vi "temp. meas. version2 v2_LV2010GF.vi"() -> ()   [LabVIEW 2010]
uses:
  Instance          15 36Saved   temp. meas. version2 v2 -jrb .vi
  Instance          16 36Saved   temp. meas. version2 v2 -jrb .vi
  Instance          17 36Saved   temp. meas. version2 v2 -jrb .vi
  Instance          18 36Saved   temp. meas. version2 v2 -jrb .vi
  Instance          19 36Saved   temp. meas. version2 v2 -jrb .vi
  Instance          20 36Saved   temp. meas. version2 v2 -jrb .vi
  <vilib>/Utility/file.llb/Read From Spreadsheet File (DBL).vi
  Instance           9 36Saved   temp. meas. version2 v2 -jrb .vi
  Instance          10 36Saved   temp. meas. version2 v2 -jrb .vi
  Instance          11 36Saved   temp. meas. version2 v2 -jrb .vi
  Instance          12 36Saved   temp. meas. version2 v2 -jrb .vi
  Instance          13 36Saved   temp. meas. version2 v2 -jrb .vi
  Instance          14 36Saved   temp. meas. version2 v2 -jrb .vi
  <vilib>/Utility/file.llb/Write To Spreadsheet File (DBL).vi
  <vilib>/Analysis/NI_AALBase.lvlib
panel:
  in  "Read Volt From Pi":bool=TRUE
  out "Voltage":string
  out "RPi temp2":string
  out "RPi Top Temp":string
  in  "Port":dbl=8901.0
  in  "IP Address":string="152.1.52.40"
  in  "Read Temp From Pi":bool=TRUE
  out "Laser Amp. Graph":cluster{"all rows":dbl[], "all rows":dbl[]}[](graph)=[{"all rows"=[32.91406, 52.36328, 73.22656, 93.29297, 112.7578], "all rows"=[-0.4725, -0.465, -0.4825, -0.485, -0.49]}]
  out "Paused":bool
  in  "NOTES":string
  in  "PAUSE next quasi wattime":bool
  in  "Num points to sum":i32=4
  out "Tive Vs Quasi-waittime*->":cluster{dbl[], dbl[]}[](graph)
  in  "PAUSE next ratio":bool
  in  "manually added info":T1
  out "lockin units":string
  out "Time v. counts/Las.Amp Graph":cluster{"all rows":dbl[], "all rows":dbl[]}[](graph)=[{"all rows"=[32.91406, 52.36328, 73.22656, 93.29297, 112.7578], "all rows"=[4.0, inf, -1.0, nan, 2.0]}]
  out "Gabes std (counter":dbl=nan format="%.3e"
  in  "Lockin settings":T2={"slope"=1, "Input Mode"=0, "time constant"=6, "display type"=1, "Range"=7, "Line reject"=1, "Filter Type"=0, "Auto freq tuning"=TRUE, "Filter Frequency (Hz)"=1000.0, "Auto Sensitivity"=FALSE, "Auto Measure"=FALSE, "Auto Phase"=TRUE} {"Filter Frequency (Hz)" min=2.0 max=1250000.0 step=1.0; "Filter Type" items=["Flat", "Notch", "Low-Pass", "Bandpass"]; "Line reject" items=["OFF", "2F", "F", "F & 2F"]; "Range" items=["100 nV", "300 nV", "1 uV", "3 uV", "10 uV", "30 uV", "100 uV", "300 uV", "1 mV", "3 mV", "10 mV", "30 mV", "100 mV", "300 mV", "1 V", "3 V"]; "display type" items=["Output %", "Output calibrated ", "Ratio", "log Ratio", "ADC 1", "ADC 2", " ADC 3", "ADC 4", "Noise %", "Noise Calibrated", "Ref. Frequency"]; "time constant" items=["1 ms", "3 ms", "10 ms", "30 ms", "100 ms", "300 ms", "1 s", "3 s", "10 s", "30 s", "100 s", "300 s", "1 ks", "3 ks"]; "Input Mode" items=["Voltage Input ( A or A-B)", "Current Input 10E6 V/A", "Current Input 10E8 V/A"]; "slope" items=["6dB/octave", "12dB/octave"]}
  out "Extra Steps taken DOWN":dbl
  out "Extra Steps taken UP":dbl
  in  "Extra steps on way TO TROUGH":dbl
  in  "extra steps on way TO PEAK":dbl
  out "peak loop counter":u32=1
  out "trough loop counter":u32=1
  out "lockin peak std":dbl=0.0050000000000000044
  out "lockin peak avg.":dbl=-0.495
  out "cB peak std":dbl=0.5
  out "cB peak avg.":dbl=0.5
  out "cA peak std":dbl
  out "cA peak avg.":dbl
  out "lockin  trough std":dbl=0.0050000000000000044
  out "lockin  trough avg.":dbl=-0.485
  out "cB trough std":dbl=1.0
  out "cB  trough avg":dbl=1.0
  out "cA trough std":dbl
  out "cA trough avg.":dbl
  in  "(m) # measurements \npe r wavelength":dbl=1.0 format="%#_2f"
  out "Time v. Ratio Graph":cluster{"all rows":dbl[], "all rows":dbl[]}[](graph)=[{"all rows"=[32.91406, 52.36328, 73.22656, 93.29297, 112.7578], "all rows"=[4.0, inf, -1.0, nan, 2.0]}]
  in  "Current Wavelength (nm)":dbl=475.0
  in  "GPIB Address SR400":string="0:23"
  in  "File name (all data)":string="temp_stats.txt"
  in  "File path":path=path "C:/users/Data/fluorescence"
  out "Ratio (counter)":dbl=2.0 format="%.3e"
  out "std (counter)":dbl=nan format="%.3e"
  out "std":dbl=4.817177617164692 format="%.3e"
  out "Time":dbl=112.7578125 format="%.3e"
  out "meas. loop counter (0 to n-1)":u32=4
  in  "# Temp. Meas. (n)":i32=10000
  out "std (lockin)":dbl=-0.00500078099915926 format="%.2f"
  out "Laser Amp. (lockin)":dbl=-0.49 format="%.3e"
  out "peak wavelength":i32=474 format="%.1f"
  out "peak lockin":dbl=-0.5 format="%.4e"
  out "peak counter B":dbl format="%.4e"
  out "peak counter A":dbl format="%.4e"
  in  "Start Wavelength (nm)":dbl=475.0
  out "trough wavelength":i32=460 format="%.1f"
  out "trough lockin":dbl=-0.48 format="%.4e"
  out "trough counter B":dbl format="%.4e"
  out "trough counter A":dbl format="%.4e"
  in  "Mode Control":T3(ring)
  in  "Wait Time (s)":dbl=5.0
  in  "Peak Wavelength (nm)":dbl=475.0
  in  "Trough Wavelength (nm)":dbl=465.0
  out "Wavelength Range Warning":bool
  in  "GPIB Address Lock-In":u8=12 min=1 max=32 step=1
  in  "GPIB Address OSC (GPIB[1]::4)":string="GPIB0::4"
  in  "Parallel Port Address":i16=888 format="%.0x"
  # "GABRIELS VARIANT OF Temperature Fluorescence Measurement"
  # "This program uses the first GPIB board (GPIB0)\ndefault addresses:\n     monochromator   x378 (parallel port)\n     lockin  GPIB0::12 (hardwired\n     osc      GPIB0::4 (not used)\n     counter 0:23"
  # "Oscilloscope Setup\n(TEKTRONIX TDS 420)"
  # "Photon Counter Setup\n(SRS 400)"
  # "Monochromator Setup\n(SPEX 1680B)"
  # "Lock-In Setup\n(EG&G 5209)"
  # "Perylene**: wavelength pairs: literature 464/476 nm \n                                             measured*: 460/475 nm\n                       ckc measured (Mar 2014): 464/476 nm"
  # "Gabes Variant"
  # "LAST DATA POINT"
  # "LAST TEMP. MEASUREMENT"
  # "**  A. J. Bur, M. G. Vangel, and S. Roth \"Temperature Dependence of Fluorescent Probes\nfor Applications to Polymer Materials Processing,\" Appl. Spec. 56, 174 (2002)."
  # "EG&G 5209 Lockin Amplifier:\n1. Manually set appropriate front\npanel settings (Sensitivity, Filters,\nand Phase).\n2. Set Time Constant to be appropriate for\nthe given REF FREQ and Wait Time (used\nabove)."
  # "SR400 Photon Counter:\n1. Run photon counter vi\nor manually control desired\nsettings.\n2. Set Wait Time to Tpreset\n3. Run this program."
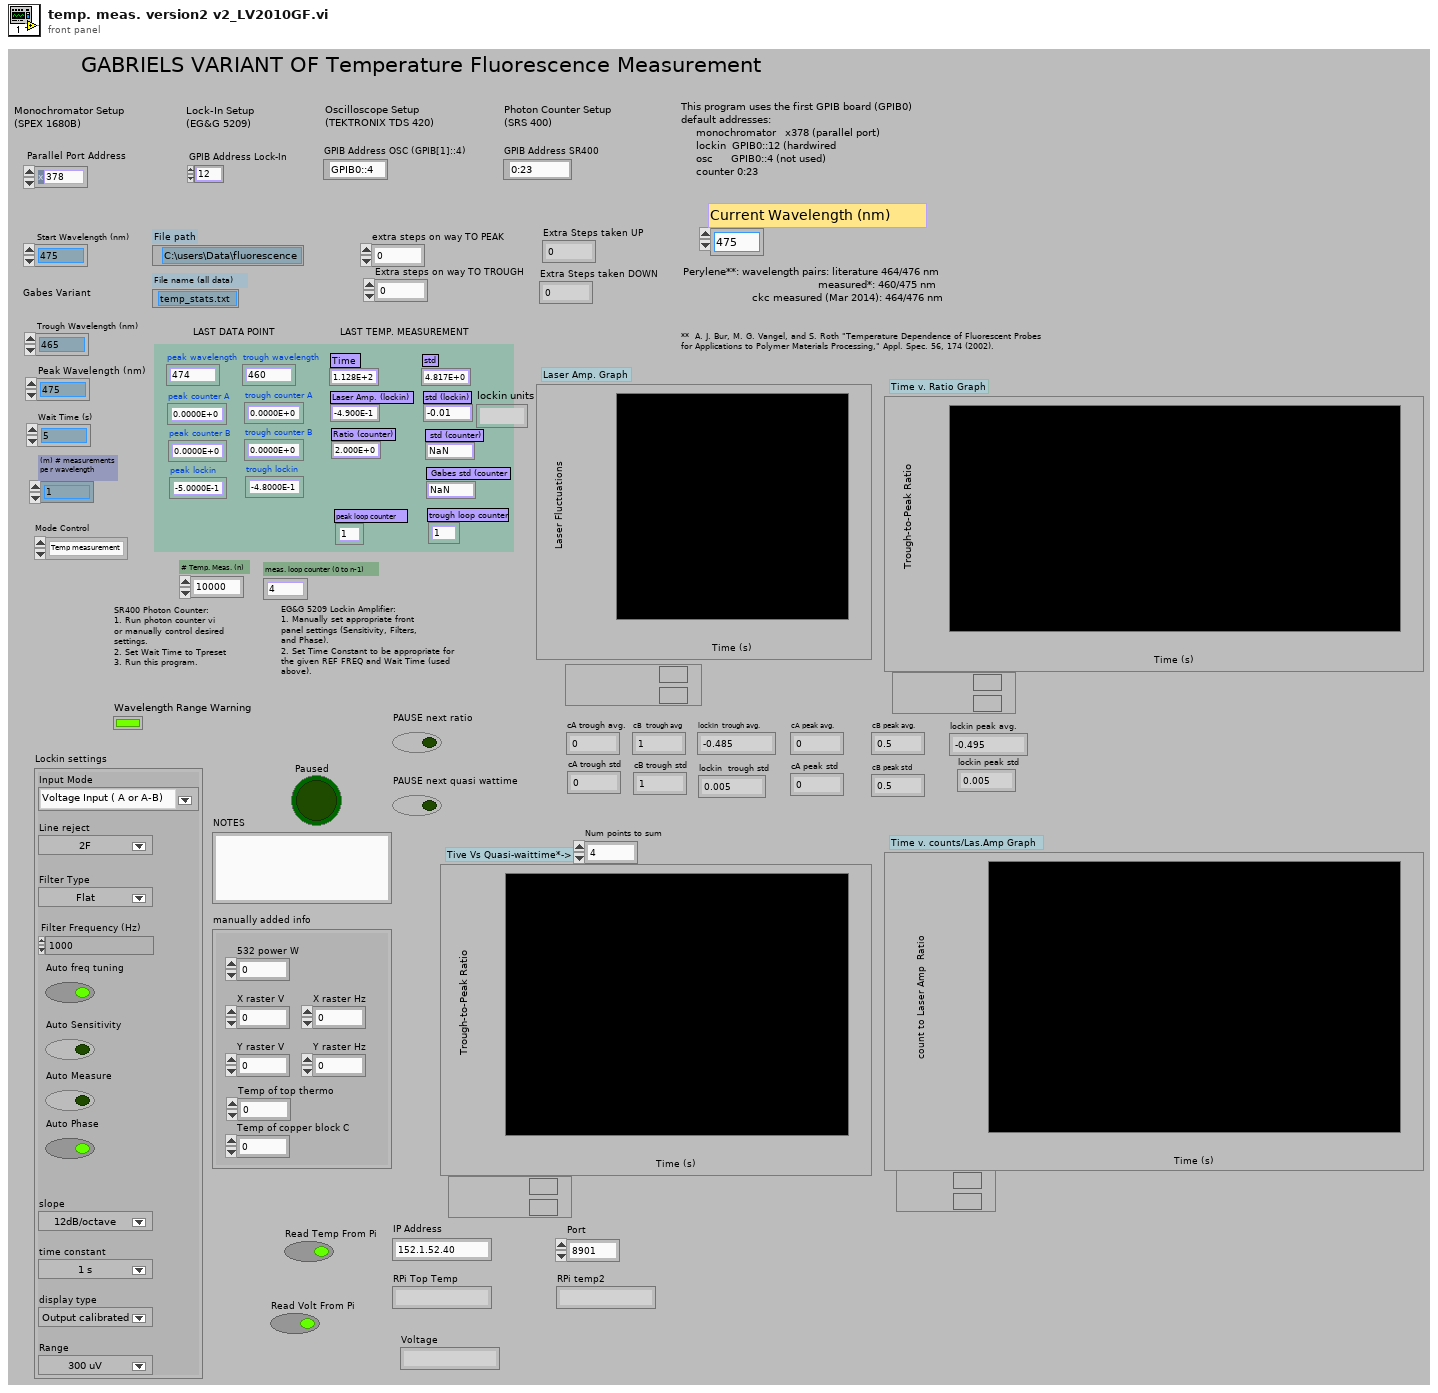
[diagram p1: front panel]
types:
  T1 = cluster{"532 power W":dbl, "X raster V":dbl, "X raster Hz ":dbl, "Y raster V":dbl, "Y raster Hz":dbl, "Temp of copper block C":dbl, "Temp of top thermo":dbl}
  T2 = cluster{"slope":i32, "Input Mode":i32, "time constant":i32, "display type":i32, "Range":i32, "Line reject":i32, "Filter Type":i32, "Auto freq tuning":bool, "Filter Frequency (Hz)":dbl, "Auto Sensitivity":bool, "Auto Measure":bool, "Auto Phase":bool}
  T3 = enum32{"Temp measurement", "Temperature Measurement"}
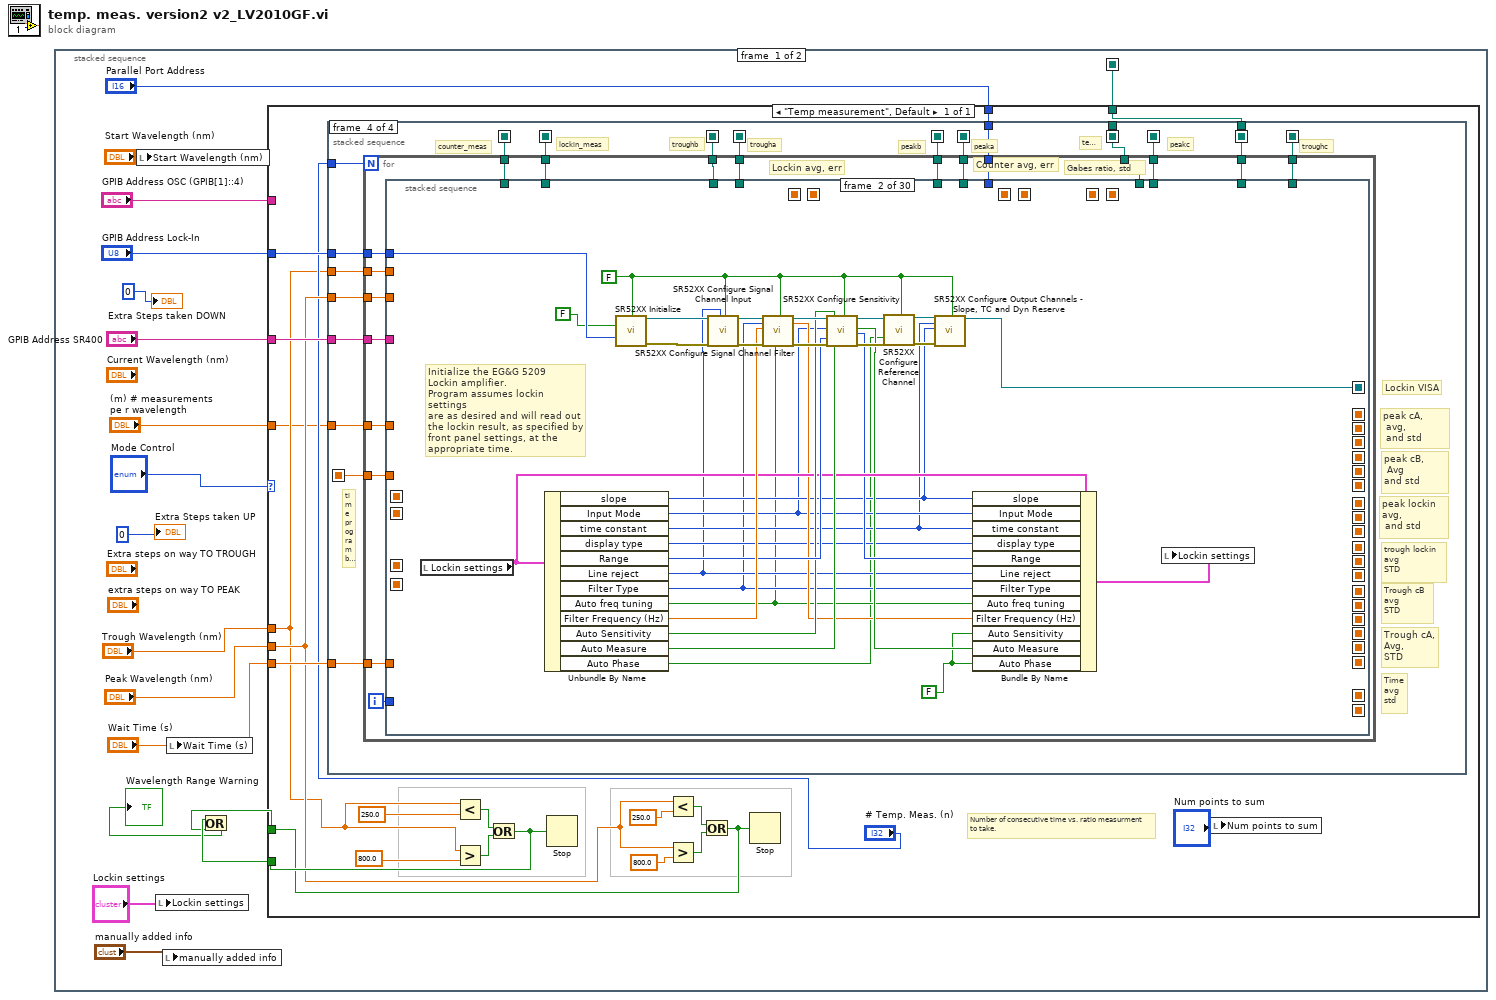
[diagram p0: block diagram]
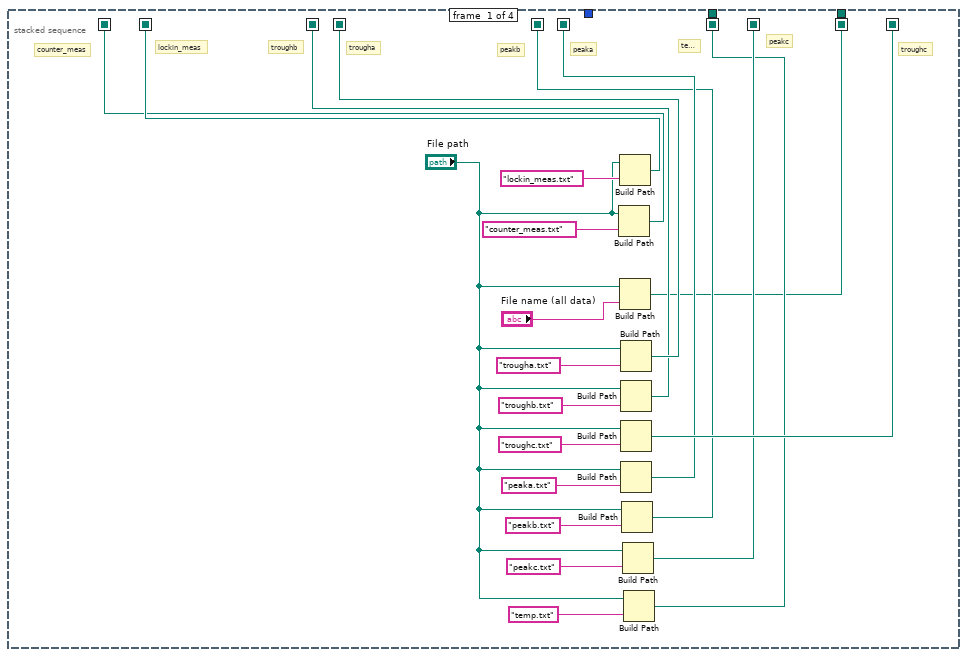
[diagram p2: hidden frame]
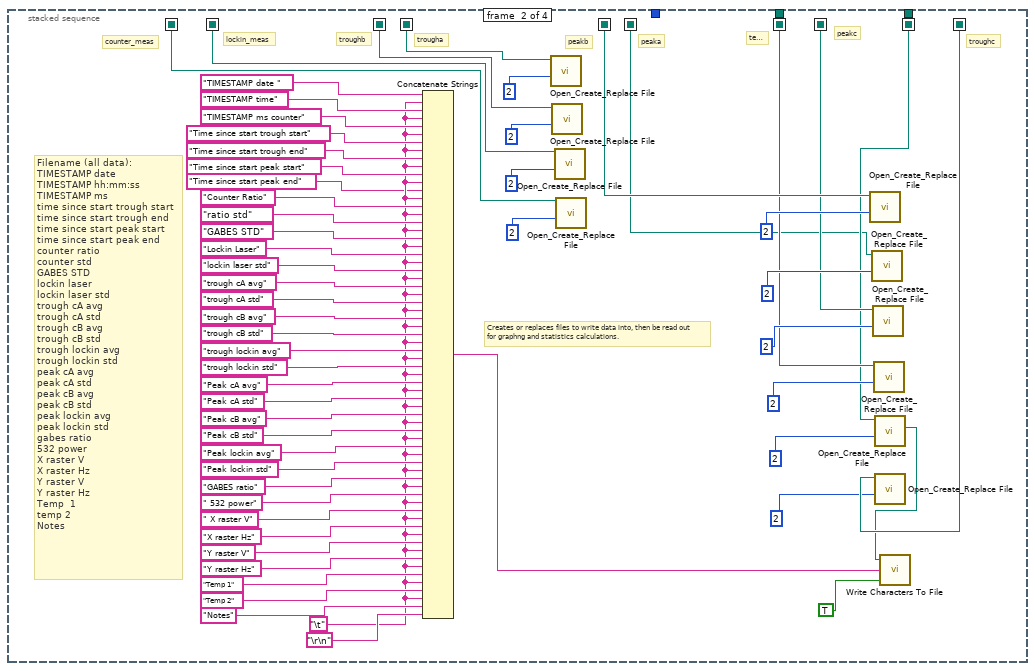
[diagram p3: hidden frame]
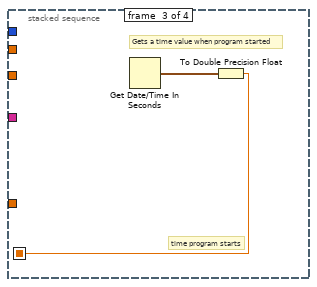
[diagram p4: hidden frame]
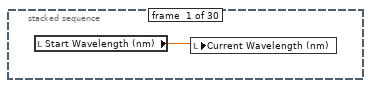
[diagram p5: hidden frame]
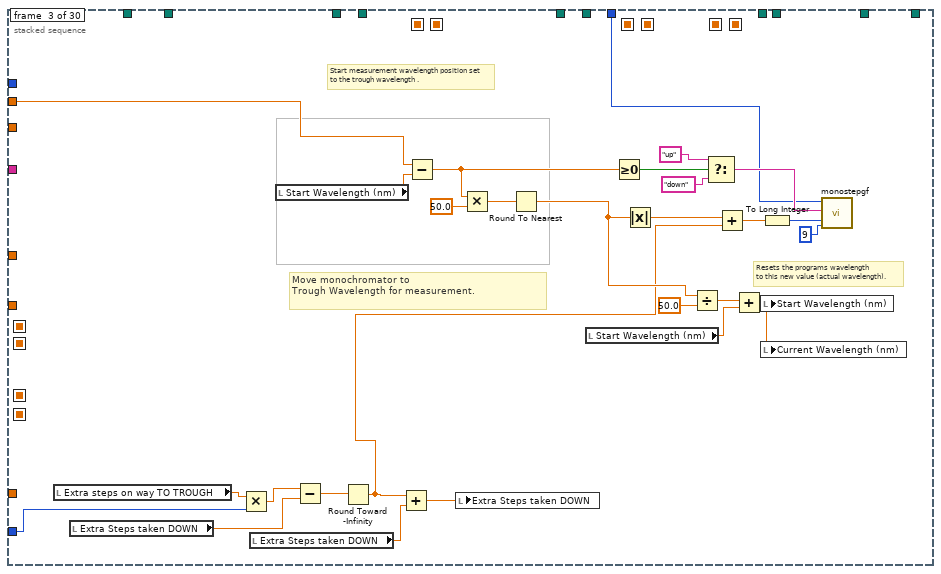
[diagram p6: hidden frame]
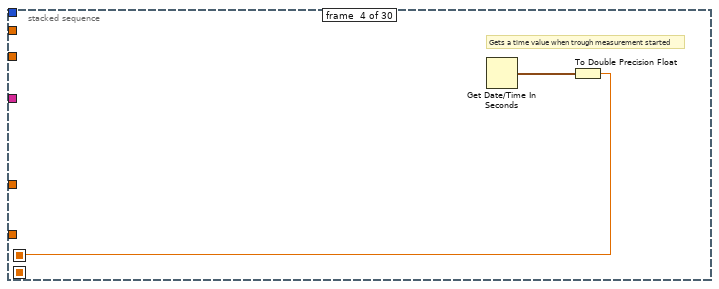
[diagram p7: hidden frame]
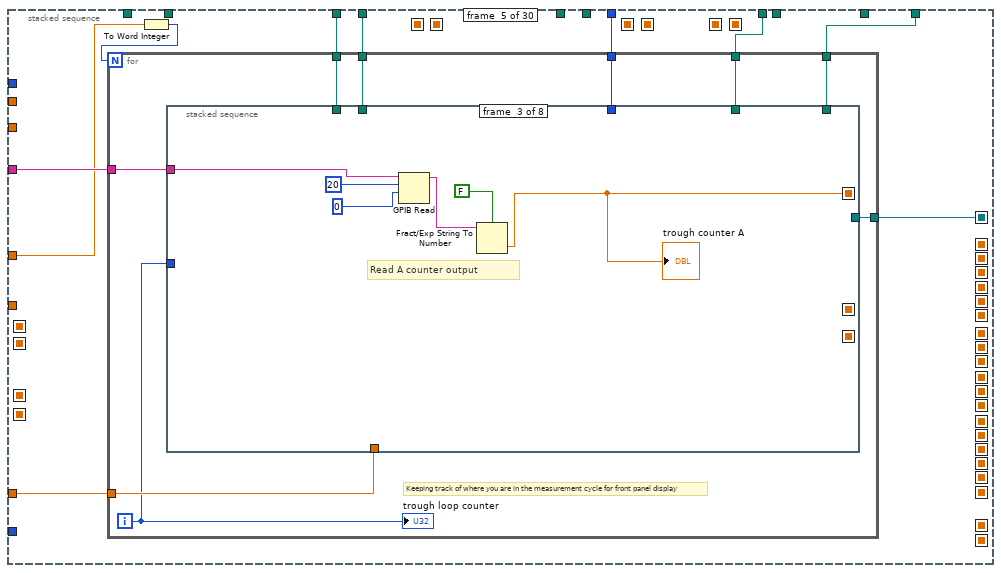
[diagram p8: hidden frame]
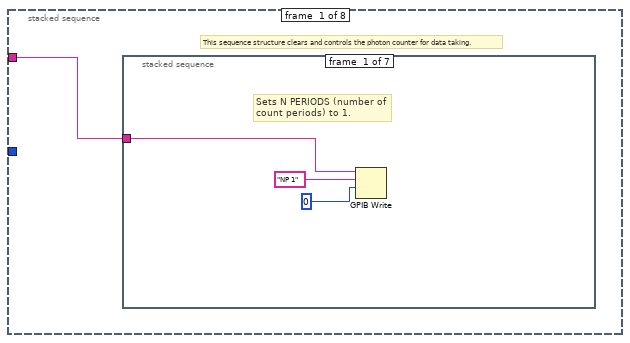
[diagram p9: hidden frame]
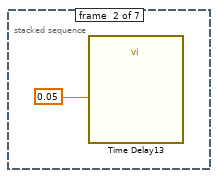
[diagram p10: hidden frame]
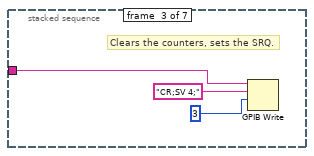
[diagram p11: hidden frame]
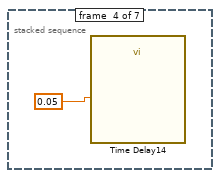
[diagram p12: hidden frame]
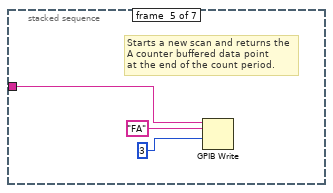
[diagram p13: hidden frame]
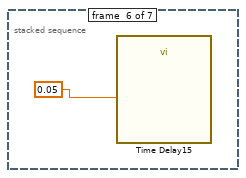
[diagram p14: hidden frame]
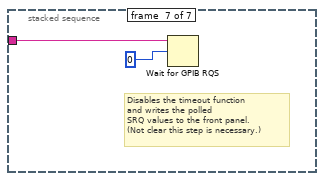
[diagram p15: hidden frame]
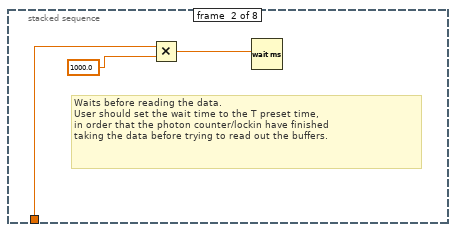
[diagram p16: hidden frame]
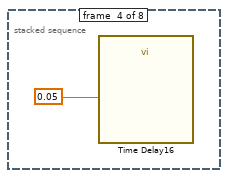
[diagram p17: hidden frame]
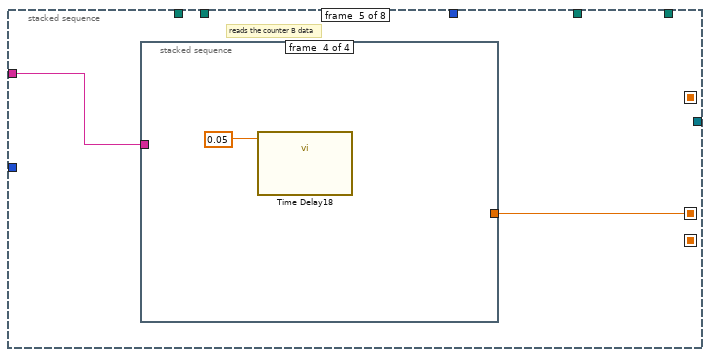
[diagram p18: hidden frame]
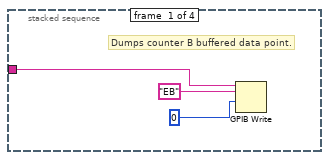
[diagram p19: hidden frame]
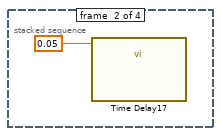
[diagram p20: hidden frame]
diagram:
  n1 = stacked-sequence {
    seq-local: [w10 _] -> [_ w887]
    frame #0 {
      n2 = local write "Start Wavelength (nm)"("Start Wavelength (nm)") -> ()
      n3 = local write "Lockin settings"("Lockin settings") -> ()
      n4 = local write "manually added info"("manually added info") -> ()
      n5 = local write "Wait Time (s)"("Wait Time (s)") -> ()
      n6 = case shown="\"Temp measurement\", Default" "Mode Control" {
        tunnel: "Parallel Port Address" -> [w30]
        tunnel: "GPIB Address OSC (GPIB[1]::4)" -> [_]
        tunnel: [w26] -> w16
        tunnel: [w24] -> w15
        tunnel: "GPIB Address Lock-In" -> [w27]
        tunnel: "GPIB Address SR400" -> [w29]
        tunnel: "Peak Wavelength (nm)" -> [w25]
        tunnel: "Trough Wavelength (nm)" -> [w22]
        tunnel: "Wait Time (s)" -> [w28]
        tunnel: [w20] -> w10
        tunnel: "(m) # measurements \npe r wavelength" -> [w21]
        frame "Temp measurement", Default {
          # "Number of consecutive time vs. ratio measurment\nto take."
          n7 = stacked-sequence {
            seq-local: [_ _ w118 _] -> [_ _ _ w131]
            seq-local: [w59 _ _ _] -> [_ w75 _ w130]
            seq-local: [w41 _ _ _] -> [_ w104 _ w129]
            seq-local: [w50 _ _ _] -> [_ w76 _ w127]
            seq-local: [w51 _ _ _] -> [_ w73 _ w128]
            seq-local: [w49 _ _ _] -> [_ w117 _ w126]
            seq-local: [w47 _ _ _] -> [_ w107 _ w124]
            seq-local: [w48 _ _ _] -> [_ w102 _ w125]
            seq-local: [w46 _ _ _] -> [_ w105 _ w123]
            seq-local: [w44 _ _ _] -> [_ w106 _ w122]
            seq-local: [w39 _ _ _] -> [_ w74 _ w121]
            tunnel: w22 -> [_ _ _ w138]
            tunnel: w30 -> [_ _ _ w137]
            tunnel: w25 -> [_ _ _ w133]
            tunnel: w29 -> [_ _ _ w134]
            tunnel: w27 -> [_ _ _ w136]
            tunnel: w28 -> [_ _ _ w135]
            tunnel: "# Temp. Meas. (n)" -> [_ _ _ w132]
            tunnel: [w44 _ _ _] -> _
            tunnel: w21 -> [_ _ _ w120]
            tunnel: [w41 _ _ _] -> w20
            frame #0 {
              # "temp"
              # "counter_meas"
              # "lockin_meas"
              # "peakc"
              # "peakb"
              # "peaka"
              # "troughc"
              # "troughb"
              # "trougha"
              n8 = Build Path(base path="File path", name or relative path="counter_meas.txt") -> (appended path=w39:path)
              n9 = Build Path(base path="File path", name or relative path="lockin_meas.txt") -> (appended path=w59:path)
              n10 = Build Path(base path="File path", name or relative path="File name (all data)") -> (appended path=w41:path)
              n11 = Build Path(base path="File path", name or relative path="trougha.txt") -> (appended path=w51:path)
              n12 = Build Path(base path="File path", name or relative path="troughb.txt") -> (appended path=w50:path)
              n13 = Build Path(base path="File path", name or relative path="troughc.txt") -> (appended path=w49:path)
              n14 = Build Path(base path="File path", name or relative path="peaka.txt") -> (appended path=w48:path)
              n15 = Build Path(base path="File path", name or relative path="peakb.txt") -> (appended path=w47:path)
              n16 = Build Path(base path="File path", name or relative path="peakc.txt") -> (appended path=w46:path)
              n17 = Build Path(base path="File path", name or relative path="temp.txt") -> (appended path=w44:path)
            }
            frame #1 {
              w61 = "\t"
              # "temp"
              # "counter_meas"
              # "lockin_meas"
              # "peakc"
              # "peakb"
              # "peaka"
              # "troughc"
              # "troughb"
              # "trougha"
              # "Filename (all data):\nTIMESTAMP date\nTIMESTAMP hh:mm:ss\nTIMESTAMP ms\ntime since start trough start\ntime since start trough end\ntime since start peak start\ntime since start peak end\ncounter ratio\ncounter std\nGABES STD\nlockin laser\nlockin laser std\ntrough cA avg\ntrough cA std\ntrough cB avg\ntrough cB std\ntrough lockin avg\ntrough lockin std\npeak cA avg\npeak cA std\npeak cB avg\npeak cB std\npeak lockin avg\npeak lockin std\ngabes ratio\n532 power\nX raster V\nX raster Hz\nY raster V\nY raster Hz\nTemp  1\ntemp 2\nNotes"
              # "Creates or replaces files to write data into, then be read out\nfor graphng and statistics calculations."
              n18 = Concatenate Strings("TIMESTAMP date ", w61, "TIMESTAMP time", w61, "TIMESTAMP ms counter", w61, "Time since start trough start", w61, "Time since start trough end", w61, "Time since start peak start", w61, "Time since start peak end", w61, "Counter Ratio", w61, "ratio std", w61, "GABES STD", w61, "Lockin Laser", w61, "lockin laser std", w61, "trough cA avg", w61, "trough cA std", w61, "trough cB avg", w61, "trough cB std", w61, "trough lockin avg", w61, "trough lockin std", w61, "Peak cA avg", w61, "Peak cA std", w61, "Peak cB avg", w61, "Peak cB std", w61, "Peak lockin avg", w61, "Peak lockin std", w61, "GABES ratio", w61, " 532 power", w61, " X raster V", w61, "X raster Hz", w61, "Y raster V", w61, "Y raster Hz", w61, "Temp 1", w61, "Temp 2", w61, "Notes", "\r\n") -> (w83:string)
              n19 = call <vilib>:"Open_Create_Replace File.vi"("function (open:0)"=2, "file path"=w73) -> ()  [unwired: 6 in, 4 out]
              n20 = call <vilib>:"Open_Create_Replace File.vi"("function (open:0)"=2, "file path"=w76) -> ()  [unwired: 6 in, 4 out]
              n21 = call <vilib>:"Open_Create_Replace File.vi"("function (open:0)"=2, "file path"=w75) -> ()  [unwired: 6 in, 4 out]
              n22 = call <vilib>:"Open_Create_Replace File.vi"("function (open:0)"=2, "file path"=w74) -> ()  [unwired: 6 in, 4 out]
              n23 = call <vilib>:"Open_Create_Replace File.vi"("function (open:0)"=2, "file path"=w107) -> ()  [unwired: 6 in, 4 out]
              n24 = call <vilib>:"Open_Create_Replace File.vi"("function (open:0)"=2, "file path"=w102) -> ()  [unwired: 6 in, 4 out]
              n25 = call <vilib>:"Open_Create_Replace File.vi"("function (open:0)"=2, "file path"=w105) -> ()  [unwired: 6 in, 4 out]
              n26 = call <vilib>:"Open_Create_Replace File.vi"("function (open:0)"=2, "file path"=w106) -> ()  [unwired: 6 in, 4 out]
              n27 = call <vilib>:"Open_Create_Replace File.vi"("function (open:0)"=2, "file path"=w104) -> ("new file path"=w82:path)  [unwired: 6 in, 3 out]
              n28 = call <vilib>:"Open_Create_Replace File.vi"("function (open:0)"=2, "file path"=w117) -> ()  [unwired: 6 in, 4 out]
              n29 = call <vilib>:"Write Characters To File.vi"("append to file? (new file:F)"=TRUE, "character string"=w83, "file path (dialog if empty)"=w82) -> ()  [unwired: 2 in, 1 out]
            }
            frame #2 {
              # "time program starts"
              # "Gets a time value when program started"
              n30 = Get Date/Time In Seconds() -> (seconds since 1Jan1904=w119:timestamp)
              n31 = To Double Precision Float(number=w119) -> (double precision float=w118:dbl)
            }
            frame #3 {
              # "time program began"
              # "Trough cA,\nAvg,\nSTD"
              # "Time\navg\nstd"
              # "trough lockin\navg\nSTD"
              # "Trough cB\navg\nSTD"
              # "Lockin VISA"
              # "peak cB,\n Avg\nand std"
              # "peak cA,\n avg,\n and std"
              # "peak lockin  avg,\n and std"
              # "temp"
              # "counter_meas"
              # "lockin_meas"
              # "peakc"
              # "peakb"
              # "peaka"
              # "troughc"
              # "troughb"
              # "trougha"
              n32 = for {
                N: w132 -> [_]
                tunnel: w138 -> [w157]
                tunnel: w137 -> [w156]
                tunnel: w136 -> [w155]
                tunnel: w135 -> [w154]
                tunnel: w134 -> [w153]
                tunnel: w133 -> [w152]
                tunnel: w131 -> [w150]
                tunnel: w130 -> [w149]
                tunnel: w129 -> [w148]
                tunnel: w128 -> [w147]
                tunnel: w127 -> [w146]
                tunnel: w126 -> [w145]
                tunnel: w125 -> [w144]
                tunnel: w124 -> [w143]
                tunnel: w123 -> [w142]
                tunnel: w122 -> [w141]
                tunnel: w121 -> [w140]
                tunnel: w120 -> [w139]
                i -> [w151]
                # "Gabes ratio, std"
                # "Counter avg, err"
                # "Lockin avg, err"
                n33 = stacked-sequence {
                  seq-local: [_ w174 _ _ _ _ _ _ _ _ _ _ _ _ _ _ _ _ _ _ _ _ _ _ _ _ _ _ _ _] -> [_ _ _ _ w226 _ _ _ _ _ _ _ _ w427 _ _ _ _ _ _ _ _ _ _ _ _ _ _ _ w855]
                  seq-local: [_ _ _ _ _ _ _ w318 _ _ _ _ _ _ _ _ _ _ _ _ _ _ _ _ _ _ _ _ _ _] -> [_ _ _ _ _ _ _ _ _ _ _ _ _ _ _ _ _ _ _ _ _ w615 _ w660 w717 _ _ _ _ _]
                  seq-local: [_ _ _ _ _ _ _ w317 _ _ _ _ _ _ _ _ _ _ _ _ _ _ _ _ _ _ _ _ _ _] -> [_ _ _ _ _ _ _ _ _ _ _ _ _ _ _ _ _ _ _ _ _ w621 _ w661 w718 _ _ _ _ _]
                  seq-local: [_ _ _ _ _ _ _ _ w323 _ _ _ _ _ _ _ _ _ _ _ _ _ _ _ _ _ _ _ _ _] -> [_ _ _ _ _ _ _ _ _ _ _ _ _ _ _ _ _ _ _ _ _ w613 _ w659 w715 _ _ _ _ _]
                  seq-local: [_ _ _ _ _ _ _ _ w324 _ _ _ _ _ _ _ _ _ _ _ _ _ _ _ _ _ _ _ _ _] -> [_ _ _ _ _ _ _ _ _ _ _ _ _ _ _ _ _ _ _ _ _ w620 _ w658 w716 _ _ _ _ _]
                  seq-local: [_ _ _ _ _ _ _ _ _ w329 _ _ _ _ _ _ _ _ _ _ _ _ _ _ _ _ _ _ _ _] -> [_ _ _ _ _ _ _ _ _ _ _ _ _ _ _ _ _ _ _ _ w588 _ _ _ w713 _ _ _ _ _]
                  seq-local: [_ _ _ _ _ _ _ _ _ w330 _ _ _ _ _ _ _ _ _ _ _ _ _ _ _ _ _ _ _ _] -> [_ _ _ _ _ _ _ _ _ _ _ _ _ _ _ _ _ _ _ _ w587 _ _ _ w714 _ _ _ _ _]
                  seq-local: [_ _ _ _ _ _ _ _ _ _ _ _ _ _ _ _ _ _ _ w564 _ _ _ _ _ _ _ _ _ _] -> [_ _ _ _ _ _ _ _ _ _ _ _ _ _ _ _ _ _ _ _ _ _ _ _ _ _ _ _ _ _]
                  seq-local: [_ _ _ _ _ _ _ _ _ _ _ _ _ _ _ _ _ _ _ w563 _ _ _ _ _ _ _ _ _ _] -> [_ _ _ _ _ _ _ _ _ _ _ _ _ _ _ _ _ _ _ _ _ _ _ _ _ w740 _ _ _ _]
                  seq-local: [_ _ _ _ _ _ _ _ _ _ _ _ _ _ _ _ _ w553 _ _ _ _ _ _ _ _ _ _ _ _] -> [_ _ _ _ _ _ _ _ _ _ _ _ _ _ _ _ _ _ _ _ _ w619 _ w680 w707 _ _ _ _ _]
                  seq-local: [_ _ _ _ _ _ _ _ _ _ _ _ _ _ _ _ _ w552 _ _ _ _ _ _ _ _ _ _ _ _] -> [_ _ _ _ _ _ _ _ _ _ _ _ _ _ _ _ _ _ _ _ _ w623 _ w676 w708 _ _ _ _ _]
                  seq-local: [_ _ _ _ _ _ _ _ _ _ _ _ _ _ _ _ _ _ w559 _ _ _ _ _ _ _ _ _ _ _] -> [_ _ _ _ _ _ _ _ _ _ _ _ _ _ _ _ _ _ _ _ _ w617 _ w679 w709 _ _ _ _ _]
                  seq-local: [_ _ _ _ _ _ _ _ _ _ _ _ _ _ _ _ _ _ w558 _ _ _ _ _ _ _ _ _ _ _] -> [_ _ _ _ _ _ _ _ _ _ _ _ _ _ _ _ _ _ _ _ _ w622 _ w672 w710 _ _ _ _ _]
                  seq-local: [_ _ _ _ _ _ _ _ _ _ _ _ _ _ _ _ w547 _ _ _ _ _ _ _ _ _ _ _ _ _] -> [_ _ _ _ _ _ _ _ _ _ _ _ _ _ _ _ _ _ _ _ w598 _ _ _ w711 _ _ _ _ _]
                  seq-local: [_ _ _ _ _ _ _ _ _ _ _ _ _ _ _ _ w546 _ _ _ _ _ _ _ _ _ _ _ _ _] -> [_ _ _ _ _ _ _ _ _ _ _ _ _ _ _ _ _ _ _ _ w597 _ _ _ w712 _ _ _ _ _]
                  seq-local: [_ _ _ w218 _ _ _ _ _ _ _ _ _ _ _ _ _ _ _ _ _ _ _ _ _ _ _ _ _ _] -> [_ _ _ _ _ _ _ _ _ _ _ _ _ _ _ _ _ _ _ w568 _ _ _ _ w688 _ _ _ _ _]
                  seq-local: [_ _ _ _ _ _ w314 _ _ _ _ _ _ _ _ _ _ _ _ _ _ _ _ _ _ _ _ _ _ _] -> [_ _ _ _ _ _ _ _ _ _ _ _ _ _ _ _ _ _ _ w567 _ _ _ _ w687 _ _ _ _ _]
                  seq-local: [_ _ _ _ _ _ _ _ _ _ _ _ w419 _ _ _ _ _ _ _ _ _ _ _ _ _ _ _ _ _] -> [_ _ _ _ _ _ _ _ _ _ _ _ _ _ _ _ _ _ _ w566 _ _ _ _ w686 _ _ _ _ _]
                  seq-local: [_ _ _ _ _ _ _ _ _ _ _ _ _ _ w515 _ _ _ _ _ _ _ _ _ _ _ _ _ _ _] -> [_ _ _ _ _ _ _ _ _ _ _ _ _ _ _ _ _ _ _ w565 _ _ _ _ w685 _ _ _ _ _]
                  seq-local: [_ _ _ _ _ _ _ _ _ _ _ _ _ _ _ _ _ _ _ _ w589 _ _ _ _ _ _ _ _ _] -> [_ _ _ _ _ _ _ _ _ _ _ _ _ _ _ _ _ _ _ _ _ _ _ _ w734 w748 _ _ _ _]
                  seq-local: [_ _ _ _ _ _ _ _ _ _ _ _ _ _ _ _ _ _ _ _ w596 _ _ _ _ _ _ _ _ _] -> [_ _ _ _ _ _ _ _ _ _ _ _ _ _ _ _ _ _ _ _ _ _ _ _ w735 _ _ _ _ _]
                  seq-local: [_ _ _ _ _ _ _ _ _ _ _ _ _ _ _ _ _ _ _ _ _ w610 _ _ _ _ _ _ _ _] -> [_ _ _ _ _ _ _ _ _ _ _ _ _ _ _ _ _ _ _ _ _ _ _ _ w690 w742 _ _ _ _]
                  seq-local: [_ _ _ _ _ _ _ _ _ _ _ _ _ _ _ _ _ _ _ _ _ w609 _ _ _ _ _ _ _ _] -> [_ _ _ _ _ _ _ _ _ _ _ _ _ _ _ _ _ _ _ _ _ _ _ _ w732 _ _ _ _ _]
                  seq-local: [_ _ _ _ _ _ _ _ _ _ _ _ _ _ _ _ _ _ _ _ _ _ _ w678 _ _ _ _ _ _] -> [_ _ _ _ _ _ _ _ _ _ _ _ _ _ _ _ _ _ _ _ _ _ _ _ w706 _ _ _ _ _]
                  seq-local: [_ _ _ _ _ _ _ _ _ _ _ _ _ _ _ _ w545 _ _ _ _ _ _ _ _ _ _ _ _ _] -> [_ _ _ _ _ _ _ _ _ _ _ _ _ _ _ _ _ _ _ _ _ _ w644 _ _ _ _ _ _ _]
                  seq-local: [_ _ _ _ _ _ _ _ _ w328 _ _ _ _ _ _ _ _ _ _ _ _ _ _ _ _ _ _ _ _] -> [_ _ _ _ _ _ _ _ _ _ _ _ _ _ _ _ _ _ _ _ _ _ w642 _ _ _ _ _ _ _]
                  seq-local: [_ _ _ _ _ _ _ _ w322 _ _ _ _ _ _ _ _ _ _ _ _ _ _ _ _ _ _ _ _ _] -> [_ _ _ _ _ _ _ _ _ _ _ _ _ _ _ _ _ _ _ _ _ _ w645 _ _ _ _ _ _ _]
                  seq-local: [_ _ _ _ _ _ _ _ _ _ _ _ _ _ _ _ _ w551 _ _ _ _ _ _ _ _ _ _ _ _] -> [_ _ _ _ _ _ _ _ _ _ _ _ _ _ _ _ _ _ _ _ _ _ w647 _ _ _ _ _ _ _]
                  seq-local: [_ _ _ _ _ _ _ _ _ _ _ _ _ _ _ _ _ _ w557 _ _ _ _ _ _ _ _ _ _ _] -> [_ _ _ _ _ _ _ _ _ _ _ _ _ _ _ _ _ _ _ _ _ _ w646 _ _ _ _ _ _ _]
                  seq-local: [_ _ _ _ _ _ _ _ _ _ _ _ _ _ _ _ _ _ _ _ _ _ w638 _ _ _ _ _ _ _] -> [_ _ _ _ _ _ _ _ _ _ _ _ _ _ _ _ _ _ _ _ _ _ _ _ w719 w739 _ _ _ _]
                  seq-local: [_ _ _ _ _ _ _ w316 _ _ _ _ _ _ _ _ _ _ _ _ _ _ _ _ _ _ _ _ _ _] -> [_ _ _ _ _ _ _ _ _ _ _ _ _ _ _ _ _ _ _ _ _ _ w643 _ _ _ _ _ _ _]
                  tunnel: w157 -> [_ _ w202 _ _ _ _ _ _ _ _ _ _ _ _ _ _ _ _ _ _ _ _ _ _ _ _ _ _ _]
                  tunnel: w156 -> [_ _ w206 _ w227 _ _ _ _ _ _ w405 _ w428 _ _ _ _ _ _ _ _ _ _ _ _ _ _ _ _]
                  tunnel: w155 -> [_ w190 _ _ _ _ _ _ _ _ _ _ _ _ _ _ _ _ _ _ _ _ _ _ _ _ _ _ _ _]
                  tunnel: w154 -> [_ _ _ _ w229 _ _ _ _ _ _ _ _ w429 _ _ _ _ _ _ _ _ _ _ _ _ _ _ _ _]
                  tunnel: w153 -> [_ _ _ _ w228 _ _ _ _ _ _ _ _ w430 _ _ _ _ _ _ _ _ _ _ _ _ _ _ _ _]
                  tunnel: w152 -> [_ _ _ _ _ _ _ _ _ _ _ w403 _ _ _ _ _ _ _ _ _ _ _ _ _ _ _ _ _ _]
                  tunnel: w151 -> [_ _ w192 _ _ _ _ _ _ _ _ w393 _ _ _ _ _ _ _ _ w599 _ _ _ _ _ _ _ _ _]
                  tunnel: w150 -> [_ _ _ _ _ _ _ _ _ _ _ _ _ _ _ _ _ _ _ w569 _ _ _ _ w689 _ _ _ _ _]
                  tunnel: w149 -> [_ _ _ _ _ _ _ _ _ _ _ _ _ _ _ _ _ _ _ _ _ _ _ _ _ w747 _ _ _ _]
                  tunnel: w148 -> [_ _ _ _ _ _ _ _ _ _ _ _ _ _ _ _ _ _ _ _ _ _ _ _ w733 _ _ _ w797 _]
                  tunnel: w147 -> [_ _ _ _ w225 _ _ w319 _ _ _ _ _ _ _ _ _ _ _ _ _ _ _ _ _ _ _ _ _ w871]
                  tunnel: w146 -> [_ _ _ _ w224 _ _ _ w325 _ _ _ _ _ _ _ _ _ _ _ _ _ _ _ _ _ _ _ _ w870]
                  tunnel: w145 -> [_ _ _ _ w223 _ _ _ _ w331 _ _ _ _ _ _ _ _ _ _ _ _ _ _ _ _ _ _ _ w856]
                  tunnel: w144 -> [_ _ _ _ _ _ _ _ _ _ _ _ _ w426 _ _ _ w554 _ _ _ _ _ _ _ _ _ _ _ w862]
                  tunnel: w143 -> [_ _ _ _ _ _ _ _ _ _ _ _ _ w425 _ _ _ _ w560 _ _ _ _ _ _ _ _ _ _ w863]
                  tunnel: w142 -> [_ _ _ _ _ _ _ _ _ _ _ _ _ w424 _ _ w548 _ _ _ _ _ _ _ _ _ _ _ _ w857]
                  tunnel: w141 -> [_ _ _ _ w222 _ _ _ _ _ _ _ _ w423 _ _ _ _ _ _ _ _ _ _ _ _ _ _ _ _]
                  tunnel: w140 -> [_ _ _ _ _ _ _ _ _ _ _ _ _ _ _ _ _ _ _ _ _ _ _ _ _ w741 _ w759 _ _]
                  tunnel: w139 -> [_ _ _ _ w221 _ _ _ _ _ _ _ _ w422 _ _ _ _ _ _ _ _ _ _ _ _ _ _ _ _]
                  frame #0 {
                    n34 = local read "Start Wavelength (nm)"() -> (w158:dbl)
                    n35 = local write "Current Wavelength (nm)"(w158) -> ()
                  }
                  frame #1 {
                    w160 = FALSE ("reset")
                    w179 = FALSE ("reset")
                    # "Initialize the EG&G 5209\nLockin amplifier.\nProgram assumes lockin settings\nare as desired and will read out\nthe lockin result, as specified by \nfront panel settings, at the\nappropriate time."
                    n36 = local read "Lockin settings"() -> (w172:T2)
                    n37 = Unbundle By Name(w172) -> ("slope"=w168:i32, "Input Mode"=w167:i32, "time constant"=w166:i32, "display type"=w165:i32, "Range"=w177:i32, "Line reject"=w164:i32, "Filter Type"=w163:i32, "Auto freq tuning"=w162:bool, "Filter Frequency (Hz)"=w178:dbl, "Auto Sensitivity"=w175:bool, "Auto Measure"=w176:bool, "Auto Phase"=w161:bool)
                    n38 = call "SR52XX Initialize"("Interface"=FALSE, "Port"=w190, "reset"=w179) -> ("VISA session"=w189:refnum<visa-resource-name>, "error out"=w188:errorcluster)  [unwired: 10 in, 1 out]
                    n39 = call "SR52XX Configure Signal Channel Input"("VISA session (for class)"=w189, "error in (no error)"=w188, "Line Frequency Rejection Filter"=w164, "Update"=w179) -> ("VISA session"=w187:refnum<visa-resource-name>, "error out"=w185:errorcluster)  [unwired: 14 in]
                    n40 = call "SR52XX Configure Signal Channel Filter"("VISA session (for class)"=w187, "FilterType"=w163, "Filter Frequency (Hz)"=w178, "error in (no error)"=w185, "Filter Tuning"=w162, "Update"=w179) -> ("VISA session"=w186:refnum<visa-resource-name>, "Filter Frequency (Hz) out"=w169:dbl, "error out"=w184:errorcluster)  [unwired: 11 in]
                    n41 = call "SR52XX Configure Sensitivity"("VISA session (for class)"=w186, "Input Mode"=w167, "Range"=w177, "error in (no error)"=w184, "Auto Sensitivity"=w175, "Auto Measure"=w176, "Update"=w179) -> ("VISA session"=w183:refnum<visa-resource-name>, "Auto Measure out"=w170:bool, "Range Out"=w171:u8, "error out"=w182:errorcluster)  [unwired: 7 in, 2 out]
                    n42 = call "SR52XX Configure Reference Channel"("VISA session (for class)"=w183, "Auto Phase"=w161, "error in (no error)"=w182, "Update"=w179) -> ("VISA session"=w181:refnum<visa-resource-name>, "error out"=w180:errorcluster)  [unwired: 12 in, 2 out]
                    n43 = call "SR52XX Configure Output Channels - Slope, TC and Dyn Reserve"("VISA session (for class)"=w181, "Time Constant"=w166, "Slope"=w168, "error in (no error)"=w180, "Update"=w179) -> ("VISA session"=w174:refnum<visa-resource-name>)  [unwired: 11 in, 3 out]
                    n44 = Bundle By Name(cluster=w172, "slope"=w168, "Input Mode"=w167, "time constant"=w166, "display type"=w165, "Range"=w171, "Line reject"=w164, "Filter Type"=w163, "Auto freq tuning"=w162, "Filter Frequency (Hz)"=w169, "Auto Sensitivity"=w160, "Auto Measure"=w170, "Auto Phase"=w160) -> (w173:T2)
                    n45 = local write "Lockin settings"(w173) -> ()
                  }
                  frame #2 {
                    # "Resets the programs wavelength\nto this new value (actual wavelength)."
                    # "Start measurement wavelength position set\nto the trough wavelength ."
                    # "Move monochromator to \nTrough Wavelength for measurement."
                    n46 = local read "Extra steps on way TO TROUGH"() -> (w199:dbl)
                    n47 = local read "Extra Steps taken DOWN"() -> (w198:dbl)
                    n48 = Multiply(x=w199, y=w192) -> (x*y=w197:dbl)
                    n49 = local read "Extra Steps taken DOWN"() -> (w193:dbl)
                    n50 = local read "Start Wavelength (nm)"() -> (w205:dbl)
                    n51 = Subtract(x=w197, y=w198) -> (x-y=w196:dbl)
                    n52 = Round Toward -Infinity(1:w196) -> (0:w195:dbl)
                    n53 = Add(x=w195, y=w193) -> (x+y=w194:dbl)
                    n54 = Subtract(x=w202, y=w205) -> (x-y=w210:dbl)
                    n55 = local write "Extra Steps taken DOWN"(w194) -> ()
                    n56 = Multiply(x=w210, y=50.0) -> (x*y=w211:dbl)
                    n57 = Round To Nearest(number=w211) -> (nearest integer value=w207:dbl)
                    n58 = local read "Start Wavelength (nm)"() -> (w204:dbl)
                    n59 = Greater Or Equal To 0?(x=w210) -> (x >= 0?=w217:bool)
                    n60 = Absolute Value(x=w207) -> (abs(x)=w200:dbl)
                    n61 = Divide(x=w207, y=50.0) -> (x/y=w208:dbl)
                    n62 = Select(t="up", s=w217, f="down") -> (s? t:f=w213:string)
                    n63 = Add(x=w200, y=w195) -> (x+y=w201:dbl)
                    n64 = Add(x=w208, y=w204) -> (x+y=w203:dbl)
                    n65 = local write "Start Wavelength (nm)"(w203) -> ()
                    n66 = local write "Current Wavelength (nm)"(w203) -> ()
                    n67 = To Long Integer(number=w201) -> (32bit integer=w191:i32)
                    n68 = call "monostepgf.vi"("Wait Between Steps(ms)"=u32 9, "Steps"=w191, "Direction"=w213, "address"=w206) -> ()
                  }
                  frame #3 {
                    # "Gets a time value when trough measurement started"
                    n69 = Get Date/Time In Seconds() -> (seconds since 1Jan1904=w219:timestamp)
                    n70 = To Double Precision Float(number=w219) -> (double precision float=w218:dbl)
                  }
                  frame #4 {
                    n71 = To Word Integer(number=w221) -> (16bit integer=w220:i16)
                    n72 = for {
                      N: w220 -> [_]
                      tunnel: w229 -> [w238]
                      tunnel: w228 -> [w237]
                      tunnel: w226 -> [w236]
                      tunnel: w227 -> [w235]
                      tunnel: w225 -> [w234]
                      tunnel: w224 -> [w233]
                      tunnel: w223 -> [w232]
                      tunnel: w222 -> [w231]
                      i -> [w230]
                      # "Keeping track of where you are in the measurement cycle for front panel display"
                      n73 = stacked-sequence {
                        seq-local: [_ _ w257 _ _ _ _ _] -> [_ _ _ _ _ _ w290 w298]
                        seq-local: [_ _ _ _ w265 _ _ _] -> [_ _ _ _ _ _ w288 w299]
                        seq-local: [_ _ _ _ _ w278 _ _] -> [_ _ _ _ _ _ w289 w300]
                        tunnel: w230 -> [_ _ _ _ _ _ _ _]
                        tunnel: w237 -> [w239 _ w258 _ w264 _ _ _]
                        tunnel: w236 -> [_ _ _ _ _ w285 _ _]
                        tunnel: w238 -> [_ w256 _ _ _ _ _ _]
                        tunnel: w235 -> [_ _ _ _ _ _ _ _]
                        tunnel: w234 -> [_ _ _ _ _ _ _ w297]
                        tunnel: w233 -> [_ _ _ _ _ _ _ w296]
                        tunnel: w232 -> [_ _ _ _ _ _ _ w295]
                        tunnel: w231 -> [_ _ _ _ _ _ w287 _]
                        frame #0 {
                          # "This sequence structure clears and controls the photon counter for data taking."
                          n74 = stacked-sequence {
                            tunnel: w239 -> [w240 _ w244 _ w248 _ w252]
                            frame #0 {
                              # "Sets N PERIODS (number of\ncount periods) to 1."
                              n75 = GPIB Write(0:w240, 1:"NP 1", 2:0) -> ()  [unwired: 2 in, 2 out]
                            }
                            frame #1 {
                              n76 = call "Time Delay13"("Delay Time (s)"=0.05) -> ()  [unwired: 10 in, 1 out]
                            }
                            frame #2 {
                              # "Clears the counters, sets the SRQ."
                              n77 = GPIB Write(0:w244, 1:"CR;SV 4;", 2:3) -> ()  [unwired: 2 in, 2 out]
                            }
                            frame #3 {
                              n78 = call "Time Delay14"("Delay Time (s)"=0.05) -> ()  [unwired: 10 in, 1 out]
                            }
                            frame #4 {
                              # "Starts a new scan and returns the  \nA counter buffered data point\nat the end of the count period."
                              n79 = GPIB Write(0:w248, 1:"FA", 2:3) -> ()  [unwired: 2 in, 2 out]
                            }
                            frame #5 {
                              n80 = call "Time Delay15"("Delay Time (s)"=0.05) -> ()  [unwired: 10 in, 1 out]
                            }
                            frame #6 {
                              # "Disables the timeout function\nand writes the polled \nSRQ values to the front panel.\n(Not clear this step is necessary.)"
                              n81 = Wait for GPIB RQS(3:0, 4:w252) -> ()  [unwired: 1 in, 2 out]
                            }
                          }
                        }
                        frame #1 {
                          # "Waits before reading the data.\nUser should set the wait time to the T preset time,\nin order that the photon counter/lockin have finished\ntaking the data before trying to read out the buffers."
                          n82 = Multiply(x=w256, y=1000.0) -> (x*y=w254:dbl)
                          n83 = Wait (ms)(milliseconds to wait=w254) -> ()  [unwired: 1 out]
                        }
                        frame #2 {
                          # "Read A counter output"
                          n84 = GPIB Read(0:w258, 1:20, 2:0) -> (5:w259:string)  [unwired: 2 in, 2 out]
                          n85 = Fract/Exp String To Number(use system decimal point (T)=FALSE, string=w259) -> (number=w257:dbl)  [unwired: 2 in, 1 out]
                          "trough counter A" <- w257
                        }
                        frame #3 {
                          n86 = call "Time Delay16"("Delay Time (s)"=0.05) -> ()  [unwired: 10 in, 1 out]
                        }
                        frame #4 {
                          # "reads the counter B data"
                          n87 = stacked-sequence {
                            tunnel: w264 -> [w266 _ w271 _]
                            tunnel: [_ _ w270 _] -> w265
                            frame #0 {
                              # "Dumps counter B buffered data point."
                              n88 = GPIB Write(0:w266, 1:"EB", 2:0) -> ()  [unwired: 2 in, 2 out]
                            }
                            frame #1 {
                              n89 = call "Time Delay17"("Delay Time (s)"=0.05) -> ()  [unwired: 10 in, 1 out]
                            }
                            frame #2 {
                              # "Reads the B counter output"
                              n90 = GPIB Read(0:w271, 1:20, 2:0) -> (5:w272:string)  [unwired: 2 in, 2 out]
                              n91 = Fract/Exp String To Number(use system decimal point (T)=FALSE, string=w272) -> (number=w270:dbl)  [unwired: 2 in, 1 out]
                              "trough counter B" <- w270
                            }
                            frame #3 {
                              n92 = call "Time Delay18"("Delay Time (s)"=0.05) -> ()  [unwired: 10 in, 1 out]
                            }
                          }
                        }
                        frame #5 {
                          # "Read Lockin Output"
                          n93 = local read "Lockin settings"() -> (w284:T2)
                          n94 = Unbundle By Name(w284) -> ("slope"=w283:i32, "Input Mode"=w282:i32, "time constant"=w281:i32, "display type"=w280:i32, "Range"=w279:i32)
                          n95 = call "SR5209 Read Output"("VISA session (for class)"=w285, "Input Mode"=w282, "Time Constant"=w281, "Display Type"=w280, "Range"=w279, "Slope"=w283) -> ("Units"=w277:string, "Output (FP)"=w278:dbl)  [unwired: 5 in, 7 out]
                          "trough lockin" <- w278
                          n96 = local write "lockin units"(w277) -> ()
                        }
                        frame #6 {
                          # "Determines the actual\nwavelength from the\nstarting wavelength\nand the number of times \nthrough theloop, and\nthe step size."
                          # "lockin"
                          # "counter B"
                          # "counter A"
                          # "wavelength"
                          # "Write to Temp File"
                          # "Current Wavelength"
                          n97 = local read "Current Wavelength (nm)"() -> (w286:dbl)
                          "trough wavelength" <- w286
                          n98 = Build Array(w286, w290, w288, w289) -> (w292:dbl[])
                          n99 = Array To Spreadsheet String(array=w292, 3:"%e" ("format string")) -> (spreadsheet string=w291:string)  [unwired: 1 in]
                          n100 = call <vilib>:"Write Characters To File.vi"("append to file? (new file:F)"=TRUE, "character string"=w291, "file path (dialog if empty)"=w287) -> ()  [unwired: 2 in, 1 out]
                        }
                        frame #7 {
                          # "lockin data"
                          # "counter B data"
                          # "counter A data"
                          # "Writes to temporary files for later computing statistics."
                          n101 = Build Array(w299) -> (w306:dbl[])
                          n102 = Build Array(w298) -> (w310:dbl[])
                          n103 = Build Array(w300) -> (w302:dbl[])
                          n104 = Array To Spreadsheet String(array=w306, 3:"%e" ("format string")) -> (spreadsheet string=w305:string)  [unwired: 1 in]
                          n105 = Array To Spreadsheet String(array=w310, 3:"%e" ("format string")) -> (spreadsheet string=w309:string)  [unwired: 1 in]
                          n106 = Array To Spreadsheet String(array=w302, 3:"%e" ("format string")) -> (spreadsheet string=w301:string)  [unwired: 1 in]
                          n107 = call <vilib>:"Write Characters To File.vi"("append to file? (new file:F)"=TRUE, "character string"=w305, "file path (dialog if empty)"=w296) -> ()  [unwired: 2 in, 1 out]
                          n108 = call <vilib>:"Write Characters To File.vi"("append to file? (new file:F)"=TRUE, "character string"=w309, "file path (dialog if empty)"=w297) -> ()  [unwired: 2 in, 1 out]
                          n109 = call <vilib>:"Write Characters To File.vi"("append to file? (new file:F)"=TRUE, "character string"=w301, "file path (dialog if empty)"=w295) -> ()  [unwired: 2 in, 1 out]
                        }
                      }
                      "trough loop counter" <- w230
                    }
                  }
                  frame #5 {
                    # "Resets the Start Wavelength to the Current Wavelength\nso the program can correctly move to the next wavelength \nmeasurement position."
                    n110 = local read "Current Wavelength (nm)"() -> (w313:dbl)
                    n111 = local write "Start Wavelength (nm)"(w313) -> ()
                  }
                  frame #6 {
                    # "Gets a time value when trough measurement completed."
                    n112 = Get Date/Time In Seconds() -> (seconds since 1Jan1904=w315:timestamp)
                    n113 = To Double Precision Float(number=w315) -> (double precision float=w314:dbl)
                  }
                  frame #7 {
                    # "counter A data trough wavelength"
                    # "Reads data from file,\ncalculates statistics."
                    n114 = call-poly <vilib>:"Read From Spreadsheet File.vi"("transpose (no:F)"=TRUE, "file path (dialog if empty)"=w319) -> ("first row"=w316:dbl[])  [unwired: 5 in, 4 out]
                    n115 = call "Update Statistics.vi"("# of groups"=1, "Input Array"=w316) -> ("new standard deviation"=w317:dbl, "new mean"=w318:dbl)  [unwired: 2 in]
                    "cA trough avg." <- w318
                    "cA trough std" <- w317
                  }
                  frame #8 {
                    # "counter B data trough wavelength"
                    # "Reads data from file,\ncalculates statistics."
                    n116 = call-poly <vilib>:"Read From Spreadsheet File.vi"("transpose (no:F)"=TRUE, "file path (dialog if empty)"=w325) -> ("first row"=w322:dbl[])  [unwired: 5 in, 4 out]
                    n117 = call "Update Statistics.vi"("# of groups"=1, "Input Array"=w322) -> ("new standard deviation"=w324:dbl, "new mean"=w323:dbl)  [unwired: 2 in]
                    "cB  trough avg" <- w323
                    "cB trough std" <- w324
                  }
                  frame #9 {
                    # "lockin data trough wavelength"
                    # "Reads data from file,\ncalculates statistics."
                    n118 = call-poly <vilib>:"Read From Spreadsheet File.vi"("transpose (no:F)"=TRUE, "file path (dialog if empty)"=w331) -> ("first row"=w328:dbl[])  [unwired: 5 in, 4 out]
                    n119 = call "Update Statistics.vi"("# of groups"=1, "Input Array"=w328) -> ("new standard deviation"=w330:dbl, "new mean"=w329:dbl)  [unwired: 2 in]
                    "lockin  trough avg." <- w329
                    "lockin  trough std" <- w330
                  }
                  frame #10 {
                    n120 = case shown="True" "Read Temp From Pi" {
                      frame False {
                      }
                      frame True {
                        n121 = while {
                          shift-right: [w384] -> w361
                          shift-left: _ -> [w387]
                          tunnel: [w378] -> w362
                          i -> [w385]
                          stop <- w381 continue-if-true
                          n122 = local read "IP Address"() -> (w390:string)
                          n123 = local read "Port"() -> (w389:dbl)
                          n124 = call <vilib>:"Clear Errors.vi"("error in (no error)"=w387) -> ("error out"=w388:errorcluster)  [unwired: 6 in]
                          n125 = Greater Or Equal?(x=5, y=w385) -> (x >= y?=w380:bool)
                          n126 = TCP Open Connection(address=w390, remote port or service name=w389, error in (no error)=w388) -> (connection ID=w378:refnum<k5>, error out=w384:errorcluster)  [unwired: 2 in]
                          n127 = Unbundle By Name(w384) -> ("code"=w382:i32)
                          n128 = Equal?(x=w382, y=56) -> (x = y?=w379:bool)
                          n129 = And(x=w379, y=w380) -> (x .and. y?=w381:bool)
                        }
                        n130 = TCP Write(connection ID=w362, data in="tem1", error in (no error)=w361) -> (connection ID out=w358:refnum<k5>, error out=w359:errorcluster)  [unwired: 1 in, 1 out]
                        n131 = TCP Read(connection ID=w358, bytes to read=6, error in (no error)=w359, 9:5000) -> (connection ID out=w354:refnum<k5>, data out=w342:string, error out=w355:errorcluster)  [unwired: 1 in]
                        "RPi Top Temp" <- w342
                        n132 = TCP Close Connection(connection ID=w354, error in (no error)=w355) -> (error out=w343:errorcluster)  [unwired: 1 in, 1 out]
                        n133 = Fract/Exp String To Number(string=w342, default (0 dbl)=0.0) -> (number=w337:dbl)  [unwired: 2 in, 1 out]
                        n134 = flat-sequence {
                          tunnel: [w377] -> w344
                          tunnel: w343 -> [w377]
                          frame #0 {
                            n135 = Wait (ms)(milliseconds to wait=1000) -> ()  [unwired: 1 out]
                          }
                        }
                        n136 = while {
                          shift-right: [w369] -> w352
                          shift-left: w344 -> [w372]
                          tunnel: [w363] -> w353
                          i -> [w370]
                          stop <- w366 continue-if-true
                          n137 = local read "IP Address"() -> (w375:string)
                          n138 = local read "Port"() -> (w374:dbl)
                          n139 = call <vilib>:"Clear Errors.vi"("error in (no error)"=w372) -> ("error out"=w373:errorcluster)  [unwired: 6 in]
                          n140 = Greater Or Equal?(x=5, y=w370) -> (x >= y?=w365:bool)
                          n141 = TCP Open Connection(address=w375, remote port or service name=w374, error in (no error)=w373) -> (connection ID=w363:refnum<k5>, error out=w369:errorcluster)  [unwired: 2 in]
                          n142 = Unbundle By Name(w369) -> ("code"=w367:i32)
                          n143 = Equal?(x=w367, y=56) -> (x = y?=w364:bool)
                          n144 = And(x=w364, y=w365) -> (x .and. y?=w366:bool)
                        }
                        n145 = local read "manually added info"() -> (w338:T1)
                        n146 = TCP Write(connection ID=w353, data in="tem2", error in (no error)=w352) -> (connection ID out=w349:refnum<k5>, error out=w350:errorcluster)  [unwired: 1 in, 1 out]
                        n147 = TCP Read(connection ID=w349, bytes to read=6, error in (no error)=w350, 9:5000) -> (connection ID out=w345:refnum<k5>, data out=w339:string, error out=w346:errorcluster)  [unwired: 1 in]
                        "RPi temp2" <- w339
                        n148 = Fract/Exp String To Number(string=w339, default (0 dbl)=0.0) -> (number=w336:dbl)  [unwired: 2 in, 1 out]
                        n149 = Bundle By Name(cluster=w338, "Temp of top thermo"=w337, "Temp of copper block C"=w336) -> (w335:T1)
                        n150 = local write "manually added info"(w335) -> ()
                        n151 = TCP Close Connection(connection ID=w345, error in (no error)=w346) -> ()  [unwired: 1 in, 2 out]
                      }
                    }
                  }
                  frame #11 {
                    # "Resets the programs wavelength\nto this new value (actual wavelength)."
                    # "Move Monochromator to Peak Wavelength \nfor the Measurement"
                    n152 = local read "extra steps on way TO PEAK"() -> (w400:dbl)
                    n153 = local read "Extra Steps taken UP"() -> (w398:dbl)
                    n154 = Increment(x=w393) -> (x+1=w392:i32)
                    n155 = Multiply(x=w400, y=w392) -> (x*y=w399:dbl)
                    n156 = Subtract(x=w399, y=w398) -> (x-y=w397:dbl)
                    n157 = local read "Extra Steps taken UP"() -> (w395:dbl)
                    n158 = Round Toward -Infinity(1:w397) -> (0:w396:dbl)
                    n159 = local read "Start Wavelength (nm)"() -> (w410:dbl)
                    n160 = Add(x=w396, y=w395) -> (x+y=w394:dbl)
                    n161 = Subtract(x=w403, y=w410) -> (x-y=w409:dbl)
                    n162 = local write "Extra Steps taken UP"(w394) -> ()
                    n163 = Multiply(x=w409, y=50.0) -> (x*y=w417:dbl)
                    n164 = Round To Nearest(number=w417) -> (nearest integer value=w406:dbl)
                    n165 = local read "Start Wavelength (nm)"() -> (w408:dbl)
                    n166 = Greater Or Equal To 0?(x=w409) -> (x >= 0?=w416:bool)
                    n167 = Absolute Value(x=w406) -> (abs(x)=w402:dbl)
                    n168 = Divide(x=w406, y=50.0) -> (x/y=w412:dbl)
                    n169 = Select(t="up", s=w416, f="down") -> (s? t:f=w407:string)
                    n170 = Add(x=w402, y=w396) -> (x+y=w401:dbl)
                    n171 = Add(x=w412, y=w408) -> (x+y=w404:dbl)
                    n172 = local write "Start Wavelength (nm)"(w404) -> ()
                    n173 = local write "Current Wavelength (nm)"(w404) -> ()
                    n174 = To Long Integer(number=w401) -> (32bit integer=w391:i32)
                    n175 = call "monostepgf.vi"("Wait Between Steps(ms)"=u32 9, "Steps"=w391, "Direction"=w407, "address"=w405) -> ()
                  }
                  frame #12 {
                    # "Gets a time value when peak  measurement started"
                    n176 = Get Date/Time In Seconds() -> (seconds since 1Jan1904=w420:timestamp)
                    n177 = To Double Precision Float(number=w420) -> (double precision float=w419:dbl)
                  }
                  frame #13 {
                    n178 = To Word Integer(number=w422) -> (16bit integer=w421:i16)
                    n179 = for {
                      N: w421 -> [_]
                      tunnel: w430 -> [w439]
                      tunnel: w429 -> [w438]
                      tunnel: w427 -> [w437]
                      tunnel: w428 -> [w436]
                      tunnel: w426 -> [w435]
                      tunnel: w425 -> [w434]
                      tunnel: w424 -> [w433]
                      tunnel: w423 -> [w432]
                      i -> [w431]
                      n180 = stacked-sequence {
                        seq-local: [_ _ w458 _ _ _ _ _] -> [_ _ _ _ _ _ w491 w499]
                        seq-local: [_ _ _ _ w465 _ _ _] -> [_ _ _ _ _ _ w489 w500]
                        seq-local: [_ _ _ _ _ w479 _ _] -> [_ _ _ _ _ _ w490 w501]
                        tunnel: w431 -> [_ _ _ _ _ _ _ _]
                        tunnel: w436 -> [_ _ _ _ _ _ _ _]
                        tunnel: w439 -> [w440 _ w459 _ w466 _ _ _]
                        tunnel: w437 -> [_ _ _ _ _ w486 _ _]
                        tunnel: w438 -> [_ w457 _ _ _ _ _ _]
                        tunnel: w435 -> [_ _ _ _ _ _ _ w498]
                        tunnel: w434 -> [_ _ _ _ _ _ _ w497]
                        tunnel: w433 -> [_ _ _ _ _ _ _ w496]
                        tunnel: w432 -> [_ _ _ _ _ _ w488 _]
                        frame #0 {
                          # "This sequence structure clears and controls the photon counter for data taking."
                          n181 = stacked-sequence {
                            tunnel: w440 -> [w441 _ w445 _ w449 _ w453]
                            frame #0 {
                              # "Sets N PERIODS (number of\ncount periods) to 1."
                              n182 = GPIB Write(0:w441, 1:"NP 1", 2:0) -> ()  [unwired: 2 in, 2 out]
                            }
                            frame #1 {
                              n183 = call "Time Delay"("Delay Time (s)"=0.05) -> ()  [unwired: 10 in, 1 out]
                            }
                            frame #2 {
                              # "Clears the counters, sets the SRQ."
                              n184 = GPIB Write(0:w445, 1:"CR;SV 4;", 2:3) -> ()  [unwired: 2 in, 2 out]
                            }
                            frame #3 {
                              n185 = call "Time Delay2"("Delay Time (s)"=0.05) -> ()  [unwired: 10 in, 1 out]
                            }
                            frame #4 {
                              # "Starts a new scan and returns the  \nA counter buffered data point\nat the end of the count period."
                              n186 = GPIB Write(0:w449, 1:"FA", 2:3) -> ()  [unwired: 2 in, 2 out]
                            }
                            frame #5 {
                              n187 = call "Time Delay3"("Delay Time (s)"=0.05) -> ()  [unwired: 10 in, 1 out]
                            }
                            frame #6 {
                              # "Disables the timeout function\nand writes the polled \nSRQ values to the front panel.\n(Not clear this step is necessary.)"
                              n188 = Wait for GPIB RQS(3:0, 4:w453) -> ()  [unwired: 1 in, 2 out]
                            }
                          }
                        }
                        frame #1 {
                          # "Waits before reading the data.\nUser should set the wait time to the T preset time."
                          n189 = Multiply(x=w457, y=1000.0) -> (x*y=w455:dbl)
                          n190 = Wait (ms)(milliseconds to wait=w455) -> ()  [unwired: 1 out]
                        }
                        frame #2 {
                          # "Read A counter output"
                          n191 = GPIB Read(0:w459, 1:20, 2:0) -> (5:w460:string)  [unwired: 2 in, 2 out]
                          n192 = Fract/Exp String To Number(use system decimal point (T)=FALSE, string=w460) -> (number=w458:dbl)  [unwired: 2 in, 1 out]
                          "peak counter A" <- w458
                        }
                        frame #3 {
                          n193 = call "Time Delay4"("Delay Time (s)"=0.05) -> ()  [unwired: 10 in, 1 out]
                        }
                        frame #4 {
                          # "reads the counter B data"
                          n194 = stacked-sequence {
                            tunnel: w466 -> [w467 _ w472 _]
                            tunnel: [_ _ w471 _] -> w465
                            frame #0 {
                              # "Dumps counter B buffered data point."
                              n195 = GPIB Write(0:w467, 1:"EB", 2:0) -> ()  [unwired: 2 in, 2 out]
                            }
                            frame #1 {
                              n196 = call "Time Delay5"("Delay Time (s)"=0.05) -> ()  [unwired: 10 in, 1 out]
                            }
                            frame #2 {
                              # "Reads the B counter output"
                              n197 = GPIB Read(0:w472, 1:20, 2:0) -> (5:w473:string)  [unwired: 2 in, 2 out]
                              n198 = Fract/Exp String To Number(use system decimal point (T)=FALSE, string=w473) -> (number=w471:dbl)  [unwired: 2 in, 1 out]
                              "peak counter B" <- w471
                            }
                            frame #3 {
                              n199 = call "Time Delay6"("Delay Time (s)"=0.05) -> ()  [unwired: 10 in, 1 out]
                            }
                          }
                        }
                        frame #5 {
                          # "Read Lockin Output"
                          n200 = local read "Lockin settings"() -> (w485:T2)
                          n201 = Unbundle By Name(w485) -> ("slope"=w484:i32, "Input Mode"=w483:i32, "time constant"=w482:i32, "display type"=w481:i32, "Range"=w480:i32)
                          n202 = call "SR5209 Read Output"("VISA session (for class)"=w486, "Input Mode"=w483, "Time Constant"=w482, "Display Type"=w481, "Range"=w480, "Slope"=w484) -> ("Units"=→"lockin units":string, "Output (FP)"=w479:dbl)  [unwired: 5 in, 7 out]
                          "peak lockin" <- w479
                        }
                        frame #6 {
                          # "lockin"
                          # "counter B"
                          # "counter A"
                          # "wavelength"
                          # "Write to Temp File"
                          # "Current Wavelength"
                          n203 = local read "Current Wavelength (nm)"() -> (w487:dbl)
                          "peak wavelength" <- w487
                          n204 = Build Array(w487, w491, w489, w490) -> (w493:dbl[])
                          n205 = Array To Spreadsheet String(array=w493, 3:"%e" ("format string")) -> (spreadsheet string=w492:string)  [unwired: 1 in]
                          n206 = call <vilib>:"Write Characters To File.vi"("append to file? (new file:F)"=TRUE, "character string"=w492, "file path (dialog if empty)"=w488) -> ()  [unwired: 2 in, 1 out]
                        }
                        frame #7 {
                          # "Write to Temp Files for later calculating statistics graphing."
                          n207 = Build Array(w500) -> (w507:dbl[])
                          n208 = Build Array(w499) -> (w511:dbl[])
                          n209 = Build Array(w501) -> (w503:dbl[])
                          n210 = Array To Spreadsheet String(array=w507, 3:"%e" ("format string")) -> (spreadsheet string=w506:string)  [unwired: 1 in]
                          n211 = Array To Spreadsheet String(array=w511, 3:"%e" ("format string")) -> (spreadsheet string=w510:string)  [unwired: 1 in]
                          n212 = Array To Spreadsheet String(array=w503, 3:"%e" ("format string")) -> (spreadsheet string=w502:string)  [unwired: 1 in]
                          n213 = call <vilib>:"Write Characters To File.vi"("append to file? (new file:F)"=TRUE, "character string"=w506, "file path (dialog if empty)"=w497) -> ()  [unwired: 2 in, 1 out]
                          n214 = call <vilib>:"Write Characters To File.vi"("append to file? (new file:F)"=TRUE, "character string"=w510, "file path (dialog if empty)"=w498) -> ()  [unwired: 2 in, 1 out]
                          n215 = call <vilib>:"Write Characters To File.vi"("append to file? (new file:F)"=TRUE, "character string"=w502, "file path (dialog if empty)"=w496) -> ()  [unwired: 2 in, 1 out]
                        }
                      }
                      "peak loop counter" <- w431
                    }
                  }
                  frame #14 {
                    # "time value  peak measurement completed."
                    # "Gets a time value when peak measurement completed."
                    n216 = Get Date/Time In Seconds() -> (seconds since 1Jan1904=w516:timestamp)
                    n217 = To Double Precision Float(number=w516) -> (double precision float=w515:dbl)
                    n218 = case shown="True" "Read Volt From Pi" {
                      frame False {
                      }
                      frame True {
                        n219 = while {
                          shift-right: [w537] -> w529
                          shift-left: _ -> [w540]
                          tunnel: [w531] -> w530
                          i -> [w538]
                          stop <- w534 continue-if-true
                          n220 = local read "IP Address"() -> (w543:string)
                          n221 = local read "Port"() -> (w542:dbl)
                          n222 = call <vilib>:"Clear Errors.vi"("error in (no error)"=w540) -> ("error out"=w541:errorcluster)  [unwired: 6 in]
                          n223 = Greater Or Equal?(x=5, y=w538) -> (x >= y?=w533:bool)
                          n224 = TCP Open Connection(address=w543, remote port or service name=w542, error in (no error)=w541) -> (connection ID=w531:refnum<k5>, error out=w537:errorcluster)  [unwired: 2 in]
                          n225 = Unbundle By Name(w537) -> ("code"=w535:i32)
                          n226 = Equal?(x=w535, y=56) -> (x = y?=w532:bool)
                          n227 = And(x=w532, y=w533) -> (x .and. y?=w534:bool)
                        }
                        n228 = TCP Write(connection ID=w530, data in="volt", error in (no error)=w529) -> (connection ID out=w526:refnum<k5>, error out=w527:errorcluster)  [unwired: 1 in, 1 out]
                        n229 = TCP Read(connection ID=w526, bytes to read=6, error in (no error)=w527, 9:5000) -> (connection ID out=w522:refnum<k5>, data out=w521:string, error out=w523:errorcluster)  [unwired: 1 in]
                        "Voltage" <- w521
                        n230 = TCP Close Connection(connection ID=w522, error in (no error)=w523) -> ()  [unwired: 1 in, 2 out]
                        n231 = Fract/Exp String To Number(string=w521, default (0 dbl)=0.0) -> (number=w517:dbl)  [unwired: 2 in, 1 out]
                        n232 = local read "manually added info"() -> (w519:T1)
                        n233 = Bundle By Name(cluster=w519, "Y raster V"=w517) -> (w518:T1)
                        n234 = local write "manually added info"(w518) -> ()
                      }
                    }
                  }
                  frame #15 {
                    # "Resets Start Wavelength based on Current Wavelength parameter."
                    n235 = local read "Current Wavelength (nm)"() -> (w544:dbl)
                    n236 = local write "Start Wavelength (nm)"(w544) -> ()
                  }
                  frame #16 {
                    # "lockin data peak wavelength"
                    # "Reads data from file,\ncalculates statistics."
                    n237 = call-poly <vilib>:"Read From Spreadsheet File.vi"("transpose (no:F)"=TRUE, "file path (dialog if empty)"=w548) -> ("first row"=w545:dbl[])  [unwired: 5 in, 4 out]
                    n238 = call "Update Statistics.vi"("# of groups"=1, "Input Array"=w545) -> ("new standard deviation"=w546:dbl, "new mean"=w547:dbl)  [unwired: 2 in]
                    "lockin peak avg." <- w547
                    "lockin peak std" <- w546
                  }
                  frame #17 {
                    # "counter A data peak wavelength"
                    # "Reads data from file,\ncalculates statistics."
                    n239 = call-poly <vilib>:"Read From Spreadsheet File.vi"("transpose (no:F)"=TRUE, "file path (dialog if empty)"=w554) -> ("first row"=w551:dbl[])  [unwired: 5 in, 4 out]
                    n240 = call "Update Statistics.vi"("# of groups"=1, "Input Array"=w551) -> ("new standard deviation"=w552:dbl, "new mean"=w553:dbl)  [unwired: 2 in]
                    "cA peak avg." <- w553
                    "cA peak std" <- w552
                  }
                  frame #18 {
                    # "counter B data peak wavelength"
                    # "Reads data from file,\ncalculates statistics."
                    n241 = call-poly <vilib>:"Read From Spreadsheet File.vi"("transpose (no:F)"=TRUE, "file path (dialog if empty)"=w560) -> ("first row"=w557:dbl[])  [unwired: 5 in, 4 out]
                    n242 = call "Update Statistics.vi"("# of groups"=1, "Input Array"=w557) -> ("new standard deviation"=w558:dbl, "new mean"=w559:dbl)  [unwired: 2 in]
                    "cB peak avg." <- w559
                    "cB peak std" <- w558
                  }
                  frame #19 {
                    # "time program began"
                    # "average peak measurement time"
                    # "time peak measuremetnt ended"
                    # "time peak measurement started"
                    # "average trough measurement time"
                    # "time trough measurement ended"
                    # "time trough measurement started"
                    # "time measurement error"
                    # "average time measurement"
                    n243 = Subtract(x=w567, y=w568) -> (x-y=w583:dbl)
                    n244 = Subtract(x=w565, y=w566) -> (x-y=w585:dbl)
                    n245 = Divide(x=w583, y=2) -> (x/y=w573:dbl)
                    n246 = Divide(x=w585, y=2) -> (x/y=w574:dbl)
                    n247 = Power Of X(1:w574, 2:2) -> (0:w572:dbl)
                    n248 = Add(x=w566, y=w574) -> (x+y=w582:dbl)
                    n249 = Add(x=w568, y=w573) -> (x+y=w578:dbl)
                    n250 = Subtract(x=w582, y=w578) -> (x-y=w580:dbl)
                    n251 = Power Of X(1:w573, 2:2) -> (0:w571:dbl)
                    n252 = Divide(x=w580, y=2) -> (x/y=w579:dbl)
                    n253 = Add(x=w572, y=w571) -> (x+y=w570:dbl)
                    n254 = Square Root(x=w570) -> (sqrt(x)=w564:dbl)
                    "std" <- w564
                    n255 = Add(x=w578, y=w579) -> (x+y=w577:dbl)
                    n256 = Subtract(x=w577, y=w569) -> (x-y=w563:dbl)
                    "Time" <- w563
                  }
                  frame #20 {
                    # "Writes the statistics information into an array and then into a string for inputting into a file."
                    # "trough lockin avg"
                    # "trough lockin std"
                    # "peak lockin std"
                    # "peak lockin avg"
                    # "lockin error"
                    # "lockin  avg."
                    n257 = Divide(x=w587, y=w588) -> (x/y=w603:dbl)
                    n258 = Add(x=w588, y=w598) -> (x+y=w595:dbl)
                    n259 = Divide(x=w597, y=w598) -> (x/y=w602:dbl)
                    n260 = Power Of X(1:w603, 2:2) -> (0:w601:dbl)
                    n261 = Power Of X(1:w602, 2:2) -> (0:w600:dbl)
                    n262 = Divide(x=w595, y=2) -> (x/y=w589:dbl)
                    "Laser Amp. (lockin)" <- w589
                    n263 = Add(x=w601, y=w600) -> (x+y=w592:dbl)
                    n264 = Divide(x=w592, y=2) -> (x/y=w591:dbl)
                    n265 = Square Root(x=w591) -> (sqrt(x)=w590:dbl)
                    n266 = Multiply(x=w589, y=w590) -> (x*y=w596:dbl)
                    "std (lockin)" <- w596
                    "meas. loop counter (0 to n-1)" <- w599
                  }
                  frame #21 {
                    # "trough counter B std"
                    # "peak counter B std"
                    # "Trough: counter A - counter B"
                    # "Peak: counter A - counter B"
                    # "peak counter B avg"
                    # "trough counter B avg"
                    # "Writes the statistics information into an array and then into a string for inputting into a file."
                    # "trough counter A avg"
                    # "trough counter A std"
                    # "peak counter A std"
                    # "peak counter A avg"
                    # "counter  measured ratio error"
                    # "counter measured ratio"
                    n267 = Subtract(x=w615, y=w613) -> (x-y=w634:dbl)
                    n268 = Subtract(x=w619, y=w617) -> (x-y=w633:dbl)
                    n269 = Divide(x=w634, y=w633) -> (x/y=w610:dbl)
                    "Ratio (counter)" <- w610
                    n270 = Divide(x=w623, y=w619) -> (x/y=w618:dbl)
                    n271 = Divide(x=w622, y=w617) -> (x/y=w616:dbl)
                    n272 = Divide(x=w621, y=w615) -> (x/y=w614:dbl)
                    n273 = Divide(x=w620, y=w613) -> (x/y=w612:dbl)
                    n274 = Power Of X(1:w612, 2:2) -> (0:w629:dbl)
                    n275 = Power Of X(1:w614, 2:2) -> (0:w624:dbl)
                    n276 = Power Of X(1:w618, 2:2) -> (0:w628:dbl)
                    n277 = Power Of X(1:w616, 2:2) -> (0:w627:dbl)
                    n278 = Add(x=w628, y=w627) -> (x+y=w626:dbl)
                    n279 = Add(x=w624, y=w629) -> (x+y=w625:dbl)
                    n280 = Add(x=w626, y=w625) -> (x+y=w607:dbl)
                    n281 = Divide(x=w607, y=4) -> (x/y=w608:dbl)
                    n282 = Square Root(x=w608) -> (sqrt(x)=w611:dbl)
                    n283 = Multiply(x=w610, y=w611) -> (x*y=w609:dbl)
                    "std (counter)" <- w609
                  }
                  frame #22 {
                    w639 = enum16{"Sample", "Population"}."Population" ("Weighting (Sample)")
                    # "slightly adjusted counter ratio"
                    # "need to use pop b/c sample cant handle sample size of 1"
                    # "Adjust each  measurement by it's lockin value"
                    # "Peak cA\nPeak cB\npeak lockin\n\nTrough cA\nTough cB\nTrough lockin"
                    n284 = for {
                      tunnel: w647 -> [w657] mode=indexing
                      tunnel: w646 -> [w656] mode=indexing
                      tunnel: w644 -> [w652] mode=indexing
                      tunnel: w643 -> [w655] mode=indexing
                      tunnel: w645 -> [w654] mode=indexing
                      tunnel: w642 -> [w651] mode=indexing
                      tunnel: [w649] -> w641 mode=indexing
                      tunnel: [w648] -> w640 mode=indexing
                      n285 = Subtract(x=w657, y=w656) -> (x-y=w653:dbl)
                      n286 = Subtract(x=w655, y=w654) -> (x-y=w650:dbl)
                      n287 = Divide(x=w653, y=w652) -> (x/y=w648:dbl)
                      n288 = Divide(x=w650, y=w651) -> (x/y=w649:dbl)
                    }
                    n289 = call <vilib>:"Std Deviation and Variance.vi"("X"=w640, "Weighting (Sample)"=w639) -> ("mean"=w637:dbl)  [unwired: 2 out]
                    n290 = call <vilib>:"Std Deviation and Variance.vi"("X"=w641, "Weighting (Sample)"=w639) -> ("mean"=w636:dbl)  [unwired: 2 out]
                    n291 = Divide(x=w636, y=w637) -> (x/y=w638:dbl)
                  }
                  frame #23 {
                    # "trough counter B std"
                    # "peak counter B std"
                    # "Trough: counter A - counter B"
                    # "Peak: counter A - counter B"
                    # "peak counter B avg"
                    # "trough counter B avg"
                    # "Writes the statistics information into an array and then into a string for inputting into a file."
                    # "trough counter A avg"
                    # "trough counter A std"
                    # "peak counter A std"
                    # "peak counter A avg"
                    # "counter  measured ratio error"
                    n292 = Subtract(x=w660, y=w659) -> (x-y=w670:dbl)
                    n293 = Subtract(x=w680, y=w679) -> (x-y=w663:dbl)
                    n294 = Square(x=w670) -> (x^2=w662:dbl)
                    n295 = Multiply(x=w663, y=w661) -> (x*y=w667:dbl)
                    n296 = Multiply(x=w663, y=w658) -> (x*y=w666:dbl)
                    n297 = Divide(x=w676, y=w670) -> (x/y=w675:dbl)
                    n298 = Divide(x=w672, y=w670) -> (x/y=w673:dbl)
                    n299 = Divide(x=w666, y=w662) -> (x/y=w668:dbl)
                    n300 = Divide(x=w667, y=w662) -> (x/y=w669:dbl)
                    n301 = Square(x=w675) -> (x^2=w674:dbl)
                    n302 = Square(x=w673) -> (x^2=w671:dbl)
                    n303 = Square(x=w668) -> (x^2=w664:dbl)
                    n304 = Square(x=w669) -> (x^2=w665:dbl)
                    n305 = Compound Arithmetic op=ADD(w674, w671, w665, w664) -> (w677:dbl)
                    n306 = Square Root(x=w677) -> (sqrt(x)=w678:dbl)
                    "Gabes std (counter" <- w678
                  }
                  frame #24 {
                    w720 = "\t"
                    w736 = TRUE
                    # "Filename (all data):\nTIMESTAMP date\nTIMESTAMP hh:mm:ss\nTIMESTAMP ms\ntime since start trough start\ntime since start trough end\ntime since startpeak start\ntime since startpeak end\ncounter ratio\ncounter std\nGABES STD\nlockin laser\nlockin laser std\ntrough cA avg\ntrough cA std\ntrough cB avg\ntrough cB std\ntrough lockin avg\ntrough lockin std\npeak cA avg\npeak cA std\npeak cB avg\npeak cB std\npeak lockin avg\npeak lockin std\ngabes ratio\n532 power\nX raster V\nX raster Hz\nY raster V\nY raster Hz\nTemp of copper block"
                    # "lockin laser error"
                    # "lockin laser"
                    # "new suffix for\nstatistics data file"
                    n307 = Tick Count (ms)() -> (millisecond timer value=w729:u32)
                    n308 = Subtract(x=w688, y=w689) -> (x-y=w684:dbl)
                    n309 = Subtract(x=w687, y=w689) -> (x-y=w683:dbl)
                    n310 = Subtract(x=w686, y=w689) -> (x-y=w682:dbl)
                    n311 = Subtract(x=w685, y=w689) -> (x-y=w681:dbl)
                    n312 = Get Date/Time In Seconds() -> (seconds since 1Jan1904=w725:timestamp)
                    n313 = Number To Decimal String(number=w729) -> (decimal integer string=w727:string)  [unwired: 1 in]
                    n314 = String Length(string=w727) -> (length=w731:i32)
                    n315 = Get Date/Time String(seconds (now)=w725, want seconds? (F)=TRUE) -> (date string=w723:string, time string=w722:string)  [unwired: 1 in]
                    n316 = Subtract(x=w731, y=4) -> (x-y=w728:i32)
                    n317 = String Subset(string=w727, offset (0)=w728) -> (substring=w721:string)  [unwired: 1 in]
                    n318 = Build Array(w723, w720, w722, w720, w721, w720) -> (w698:string[])
                    n319 = local read "manually added info"() -> (w699:T1)
                    n320 = Unbundle By Name(w699) -> ("532 power W"=w705:dbl, "X raster V"=w704:dbl, "X raster Hz"=w703:dbl, "Y raster V"=w702:dbl, "Y raster Hz"=w701:dbl, "Temp of copper block C"=w700:dbl, "Temp of top thermo"=w691:dbl)
                    n321 = Build Array(w684, w683, w682, w681, w690, w732, w706, w734, w735, w717, w718, w715, w716, w713, w714, w707, w708, w709, w710, w711, w712, w719, w705, w704, w703, w702, w701, w700, w691) -> (w737:dbl[])
                    n322 = Array To Spreadsheet String(array=w737, 3:"%e") -> (spreadsheet string=w694:string)  [unwired: 1 in]
                    n323 = Search and Replace String(input string=w694, search string="\r\n", replace string="\t") -> (result string=w695:string)  [unwired: 5 in, 3 out]
                    n324 = Concatenate Strings(w698, w695, "NOTES", "\r\n") -> (w724:string)
                    n325 = call <vilib>:"Write Characters To File.vi"("convert eol? (no:F)"=w736, "append to file? (new file:F)"=w736, "character string"=w724, "file path (dialog if empty)"=w733) -> ()  [unwired: 1 in, 1 out]
                  }
                  frame #25 {
                    w745 = TRUE
                    w751 = TRUE
                    n326 = Build Array(w740, w742, w739) -> (w743:dbl[])
                    n327 = Array To Spreadsheet String(array=w743, 3:"%e") -> (spreadsheet string=w744:string)  [unwired: 1 in]
                    n328 = Build Array(w740, w748) -> (w749:dbl[])
                    n329 = call <vilib>:"Write Characters To File.vi"("convert eol? (no:F)"=w745, "append to file? (new file:F)"=w745, "character string"=w744, "file path (dialog if empty)"=w741) -> ()  [unwired: 1 in, 1 out]
                    n330 = Array To Spreadsheet String(array=w749, 3:"%e") -> (spreadsheet string=w750:string)  [unwired: 1 in]
                    n331 = call <vilib>:"Write Characters To File.vi"("convert eol? (no:F)"=w751, "append to file? (new file:F)"=w751, "character string"=w750, "file path (dialog if empty)"=w747) -> ()  [unwired: 1 in, 1 out]
                  }
                  frame #26 {
                  }
                  frame #27 {
                    # "time v. ratio graph"
                    n332 = call-poly <vilib>:"Read From Spreadsheet File.vi"("format (%.3f)"="%e", "file path (dialog if empty)"=w759) -> ("all rows"=w757:dbl[][])  [unwired: 5 in, 4 out]
                    n333 = Delete From Array(array=w757, index (col)=0 ("disabled index (col)")) -> (deleted portion=w753:dbl[])  [unwired: 2 in, 1 out]
                    n334 = Delete From Array(array=w757, index (col)=1 ("disabled index (col)")) -> (deleted portion=w754:dbl[])  [unwired: 2 in, 1 out]
                    n335 = Delete From Array(array=w757, index (col)=2 ("disabled index (col)")) -> (deleted portion=w756:dbl[])  [unwired: 2 in, 1 out]
                    n336 = Bundle "Bundle"("all rows"=w753, "all rows"=w754) -> (w760:cluster{"all rows":dbl[], "all rows":dbl[]})  [unwired: 1 in]
                    n337 = Bundle "Bundle"("all rows"=w753, "all rows"=w756) -> (w755:cluster{"all rows":dbl[], "all rows":dbl[]})  [unwired: 1 in]
                    n338 = Build Array(w760, w755) -> (→"Time v. Ratio Graph":cluster{"all rows":dbl[], "all rows":dbl[]}[])
                  }
                  frame #28 {
                    w783 = 1 ("disabled index (col)")
                    # "Peak lockin"
                    # "Peak Counter B"
                    # "Peak counter A"
                    # "trough Lockin"
                    # "trough counter B"
                    # "trough counter A"
                    # "Time"
                    n339 = call-poly <vilib>:"Read From Spreadsheet File.vi"("format (%.3f)"="%e", "file path (dialog if empty)"=w797) -> ("all rows"=w791:dbl[][])  [unwired: 5 in, 4 out]
                    n340 = Delete From Array(array=w791, index (col)=22 ("disabled index (col)")) -> (deleted portion=w785:dbl[])  [unwired: 2 in, 1 out]
                    n341 = Delete From Array(array=w791, index (col)=3 ("disabled index (col)")) -> (deleted portion=w790:dbl[])  [unwired: 2 in, 1 out]
                    n342 = Delete From Array(array=w791, index (col)=12 ("disabled index (col)")) -> (deleted portion=w789:dbl[])  [unwired: 2 in, 1 out]
                    n343 = Delete From Array(array=w791, index (col)=14 ("disabled index (col)")) -> (deleted portion=w788:dbl[])  [unwired: 2 in, 1 out]
                    n344 = Delete From Array(array=w791, index (col)=16 ("disabled index (col)")) -> (deleted portion=w787:dbl[])  [unwired: 2 in, 1 out]
                    n345 = Delete From Array(array=w791, index (col)=18 ("disabled index (col)")) -> (deleted portion=w786:dbl[])  [unwired: 2 in, 1 out]
                    n346 = Delete From Array(array=w791, index (col)=20 ("disabled index (col)")) -> (deleted portion=w784:dbl[])  [unwired: 2 in, 1 out]
                    n347 = Array Subset(array=w790, index=w783) -> (w767:dbl[])  [unwired: 1 in]
                    n348 = Array Subset(array=w789, index=w783) -> (w773:dbl[])  [unwired: 1 in]
                    n349 = Array Subset(array=w788, index=w783) -> (w774:dbl[])  [unwired: 1 in]
                    n350 = Array Subset(array=w787, index=w783) -> (w765:dbl[])  [unwired: 1 in]
                    n351 = Array Subset(array=w786, index=w783) -> (w775:dbl[])  [unwired: 1 in]
                    n352 = Array Subset(array=w784, index=w783) -> (w776:dbl[])  [unwired: 1 in]
                    n353 = Array Subset(array=w785, index=w783) -> (w766:dbl[])  [unwired: 1 in]
                    n354 = for {
                      tunnel: w773 -> [w854] mode=indexing
                      tunnel: w774 -> [w853] mode=indexing
                      tunnel: w765 -> [w849] mode=indexing
                      tunnel: w775 -> [w851] mode=indexing
                      tunnel: w776 -> [w852] mode=indexing
                      tunnel: w766 -> [w848] mode=indexing
                      tunnel: [w846] -> w780 mode=indexing
                      tunnel: [w845] -> w779 mode=indexing
                      n355 = Subtract(x=w851, y=w852) -> (x-y=w847:dbl)
                      n356 = Subtract(x=w854, y=w853) -> (x-y=w850:dbl)
                      n357 = Divide(x=w850, y=w849) -> (x/y=w846:dbl)
                      n358 = Divide(x=w847, y=w848) -> (x/y=w845:dbl)
                    }
                    n359 = while {
                      tunnel: w773 -> [w824]
                      tunnel: w767 -> [w826]
                      tunnel: [w807] -> w771 mode=indexing
                      tunnel: [w821] -> w772 mode=indexing
                      tunnel: w774 -> [w820]
                      tunnel: w775 -> [w819]
                      tunnel: w776 -> [w818]
                      i -> [w805]
                      stop <- w827 stop-if-true
                      w813 = 0.0
                      n360 = local read "Num points to sum"() -> (w802:i32)
                      n361 = Multiply(x=w805, y=w802) -> (x*y=w817:i32)
                      n362 = Array Subset(array=w818, index=w817, length=w802) -> (w814:dbl[])
                      n363 = Array Subset(array=w824, index=w817, length=w802) -> (w822:dbl[])
                      n364 = Array Size(array=w822) -> (size(s)=w828:i32)
                      n365 = Array Subset(array=w819, index=w817, length=w802) -> (w815:dbl[])
                      n366 = Array Subset(array=w826, index=w817, length=w802) -> (w825:dbl[])
                      n367 = Array Subset(array=w820, index=w817, length=w802) -> (w816:dbl[])
                      n368 = Less?(x=w828, y=w802) -> (x < y?=w827:bool)
                      n369 = for {
                        tunnel: w825 -> [w844] mode=indexing
                        shift-right: [w843] -> w823
                        shift-left: w813 -> [w842]
                        tunnel: w822 -> [w841] mode=indexing
                        shift-right: [w840] -> w812
                        shift-left: w813 -> [w839]
                        tunnel: w816 -> [w833] mode=indexing
                        tunnel: w815 -> [w834] mode=indexing
                        tunnel: w814 -> [w835] mode=indexing
                        shift-right: [w832] -> w811
                        shift-left: w813 -> [w836]
                        shift-right: [w831] -> w810
                        shift-left: w813 -> [w837]
                        shift-right: [w830] -> w809
                        shift-left: w813 -> [w838]
                        tunnel: [w829] -> w804
                        i -> [w829]
                        n370 = Add(x=w834, y=w837) -> (x+y=w831:dbl)
                        n371 = Add(x=w841, y=w839) -> (x+y=w840:dbl)
                        n372 = Add(x=w833, y=w836) -> (x+y=w832:dbl)
                        n373 = Add(x=w835, y=w838) -> (x+y=w830:dbl)
                        n374 = Add(x=w844, y=w842) -> (x+y=w843:dbl)
                      }
                      n375 = Increment(x=w804) -> (x+1=w803:i32)
                      n376 = Divide(x=w823, y=w803) -> (x/y=w821:dbl)
                      n377 = Subtract(x=w812, y=w811) -> (x-y=w808:dbl)
                      n378 = Subtract(x=w810, y=w809) -> (x-y=w806:dbl)
                      n379 = Divide(x=w808, y=w806) -> (x/y=w807:dbl)
                    }
                    n380 = Bundle "Bundle"(w767, w780) -> (w798:cluster{dbl[], dbl[]})  [unwired: 1 in]
                    n381 = Bundle "Bundle"(w767, w779) -> (w782:cluster{dbl[], dbl[]})  [unwired: 1 in]
                    n382 = Bundle "Bundle"(w767, w766) -> (w768:cluster{dbl[], dbl[]})  [unwired: 1 in]
                    n383 = Bundle "Bundle"(w767, w765) -> (w769:cluster{dbl[], dbl[]})  [unwired: 1 in]
                    n384 = Build Array(w798, w782) -> (→"Time v. counts/Las.Amp Graph":cluster{dbl[], dbl[]}[])
                    n385 = Build Array(w768, w769) -> (→"Laser Amp. Graph":cluster{dbl[], dbl[]}[])
                    n386 = Bundle "Bundle"(w772, w771) -> (w778:cluster{dbl[], dbl[]})  [unwired: 1 in]
                    n387 = Build Array(w778) -> (→"Tive Vs Quasi-waittime*->":cluster{dbl[], dbl[]}[])
                  }
                  frame #29 {
                    # "Deletes temporary files used to carry data of the\ntrough and peak wavelength measurement (counter A, counter B, and lockin) for this\ndata point (usually 3 points), so that the next\ntemperature measurement point doesn't use\nappended values."
                    n388 = while {
                      stop <- w874 continue-if-true
                      n389 = local read "Num points to sum"() -> (w879:i32)
                      n390 = local read "meas. loop counter (0 to n-1)"() -> (w880:u32)
                      n391 = Wait (ms)(milliseconds to wait=500) -> ()  [unwired: 1 out]
                      n392 = Increment(x=w880) -> (x+1=w875:u32)
                      n393 = Quotient & Remainder(x=w875, y=w879) -> (x-y*floor(x/y)=w878:u32)  [unwired: 1 out]
                      n394 = Less?(x=w878, y=1) -> (x < y?=w876:bool)
                      n395 = And(x="PAUSE next quasi wattime", y=w876) -> (x .and. y?=w874:bool)
                      "Paused" <- w874
                      n396 = case shown="False" w874 {
                        frame False {
                        }
                        frame True {
                          w884 = 100
                          n397 = call <vilib>:"Beep.vi"("use system alert? (T)"=TRUE, "duration (msec)"=w884, "frequency (Hz)"=w884) -> ()  [unwired: 9 in]
                        }
                      }
                    }
                    n398 = while {
                      stop <- "PAUSE next ratio" continue-if-true
                      n399 = Wait (ms)(milliseconds to wait=500) -> ()  [unwired: 1 out]
                    }
                    n400 = call <vilib>:"Open_Create_Replace File.vi"("advisory dialog? (display:T)"=FALSE, "function (open:0)"=2, "file path"=w871) -> ()  [unwired: 5 in, 4 out]
                    n401 = call <vilib>:"Open_Create_Replace File.vi"("advisory dialog? (display:T)"=FALSE, "function (open:0)"=2, "file path"=w870) -> ()  [unwired: 5 in, 4 out]
                    n402 = call <vilib>:"Open_Create_Replace File.vi"("advisory dialog? (display:T)"=FALSE, "function (open:0)"=2, "file path"=w862) -> ()  [unwired: 5 in, 4 out]
                    n403 = call <vilib>:"Open_Create_Replace File.vi"("advisory dialog? (display:T)"=FALSE, "function (open:0)"=2, "file path"=w863) -> ()  [unwired: 5 in, 4 out]
                    n404 = call <vilib>:"Open_Create_Replace File.vi"("advisory dialog? (display:T)"=FALSE, "function (open:0)"=2, "file path"=w856) -> ()  [unwired: 5 in, 4 out]
                    n405 = call <vilib>:"Open_Create_Replace File.vi"("advisory dialog? (display:T)"=FALSE, "function (open:0)"=2, "file path"=w857) -> ()  [unwired: 5 in, 4 out]
                    n406 = call "SR52XX Close"("VISA session"=w855) -> ()  [unwired: 1 in, 1 out]
                  }
                }
              }
            }
          }
          n407 = Less?(x=w22, y=250.0) -> (x < y?=w36:bool)
          n408 = Greater?(x=w22, y=800.0) -> (0:w35:bool)
          n409 = Or(x=w36, y=w35) -> (x .or. y?=w26:bool)
          n410 = Stop(stop? (T)=w26) -> ()
          n411 = Less?(x=w25, y=250.0) -> (x < y?=w32:bool)
          n412 = Greater?(x=w25, y=800.0) -> (0:w31:bool)
          n413 = Or(x=w32, y=w31) -> (x .or. y?=w24:bool)
          n414 = Stop(stop? (T)=w24) -> ()
          n415 = local write "Num points to sum"("Num points to sum") -> ()
        }
      }
      n416 = Or(x=w16, y=w15) -> (x .or. y?=→"Wavelength Range Warning":bool)
      "Extra Steps taken UP" <- 0
      "Extra Steps taken DOWN" <- 0
    }
    frame #1 {
      # "Save Data to File"
      n417 = Two Button Dialog(message="Would you like to save the data?", 1:"Don't Save" ("F button name (\"Cancel\")"), 2:"Save" ("T button name (\"OK\")")) -> (T button?=w888:bool)
      n418 = case shown="True" w888 {
        tunnel: w887 -> [_ w892]
        frame False {
        }
        frame True {
          n419 = stacked-sequence {
            seq-local: [w894 _] -> [_ w896]
            tunnel: w892 -> [w893 _]
            frame #0 {
              n420 = call-poly <vilib>:"Read From Spreadsheet File.vi"("format (%.3f)"="%e", "file path (dialog if empty)"=w893) -> ("all rows"=w894:dbl[][])  [unwired: 5 in, 4 out]
            }
            frame #1 {
              n421 = call-poly <vilib>:"Write To Spreadsheet File.vi"("format (%.3f)"="%e", "2D data"=w896) -> ()  [unwired: 6 in, 1 out]
            }
          }
        }
      }
    }
  }
